vi "数据表比对.vi"(8 "error in (no error)":errorcluster, 9 "查询元素输入":string(combo), 10 "仪器日志参数":string, 11 "table输入":string(combo)) -> (0 "error out":errorcluster, 1 "columns输出":string[](array[string]), 2 "待发送第一条数据":string[](array[string]), 3 "待发送数据":string[][](table))   [LabVIEW 2016, in "数据传输系统-03.lvlib"]
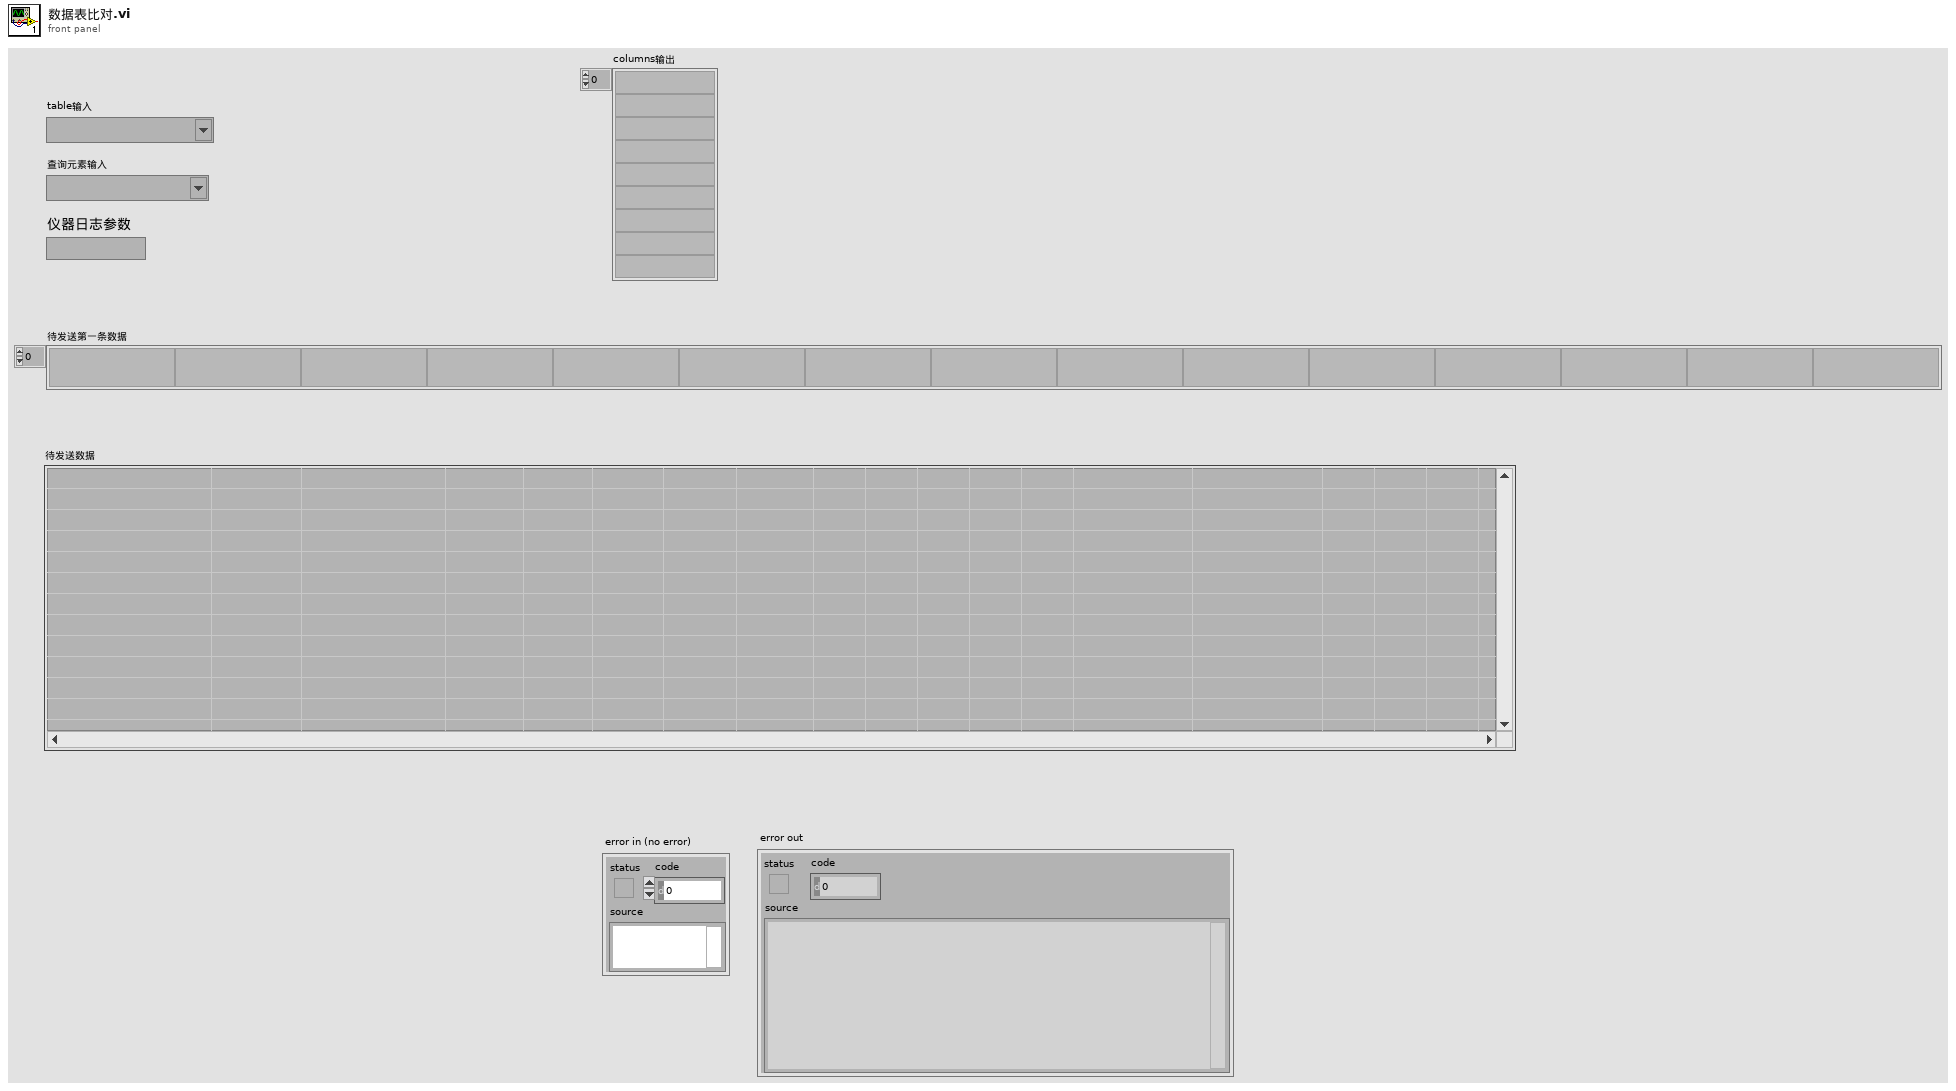
[diagram p1: front panel]
types:
  T1 = cluster{"氨氮仪器日志索引起始时间":string, "总磷仪器日志索引起始时间":string, "总氮仪器日志索引起始时间":string, "CODMn仪器日志索引起始时间":string, "CODCr仪器日志索引起始时间":string, "系统仪器日志索引起始时间":string, "氟化物仪器日志索引起始时间":string, "挥发酚仪器日志索引起始时间":string}
  T2 = cluster{"氨氮仪器参数索引起始时间":string, "总磷仪器参数索引起始时间":string, "总氮仪器参数索引起始时间":string, "CODMn仪器参数索引起始时间":string, "CODCr仪器参数索引起始时间":string, "DO仪器参数索引起始时间":string, "PH仪器参数索引起始时间":string, "比电导率仪器参数索引起始时间":string, "水温仪器参数索引起始时间":string, "浊度仪器参数索引起始时间":string, "叶绿素a仪器参数索引起始时间":string, "藻密度仪器参数索引起始时间":string, "ORP仪器参数索引起始时间":string, "氟化物仪器参数索引起始时间":string, "挥发酚仪器参数索引起始时间":string}
  T3 = typedef "数据传输系统-03.lvlib/应用环境.ctl" = enum16{"STD", "GB212", "婉仪平台"}
  T4 = cluster{"氨氮报警信息索引起始时间":string, "总磷报警信息索引起始时间":string, "总氮报警信息索引起始时间":string, "CODMn报警信息索引起始时间":string, "CODCr报警信息索引起始时间":string, "DO报警信息索引起始时间":string, "PH报警信息索引起始时间":string, "比电导率报警信息索引起始时间":string, "水温报警信息索引起始时间":string, "浊度报警信息索引起始时间":string, "叶绿素报警信息索引起始时间":string, "系统报警信息索引起始时间":string, "氟化物报警信息索引起始时间":string, "挥发酚报警信息索引起始时间":string}
  T5 = cluster{"氨氮零点核查索引起始时间":string, "总磷零点核查索引起始时间":string, "总氮零点核查索引起始时间":string, "CODMn零点核查索引起始时间":string, "CODCr零点核查索引起始时间":string, "亚硝酸盐零点核查索引起始时间":string, "硫化物零点核查索引起始时间":string, "ORP零点核查索引起始时间":string, "氟化物零点核查索引起始时间":string, "挥发酚零点核查索引起始时间":string}
  T6 = cluster{"氨氮标样核查索引起始时间":string, "总磷标样核查索引起始时间":string, "总氮标样核查索引起始时间":string, "CODMn标样核查索引起始时间":string, "CODCr标样核查索引起始时间":string, "DO标样核查索引起始时间":string, "PH标样核查索引起始时间":string, "比电导率标样核查索引起始时间":string, "水温标样核查索引起始时间":string, "浊度标样核查索引起始时间":string, "叶绿素a标样核查索引起始时间":string, "藻密度标样核查索引起始时间":string, "亚硝酸盐标样核查索引起始时间":string, "硫化物标样核查索引起始时间":string, "ORP标样核查索引起始时间":string, "氟化物标样核查索引起始时间":string, "挥发酚标样核查索引起始时间":string, "氯化物标样核查索引起始时间":string}
  T7 = cluster{"氨氮跨度核查索引起始时间":string, "总磷跨度核查索引起始时间":string, "总氮跨度核查索引起始时间":string, "CODMn跨度核查索引起始时间":string, "CODCr跨度核查索引起始时间":string, "亚硝酸盐跨度核查索引起始时间":string, "硫化物跨度核查索引起始时间":string, "ORP跨度核查索引起始时间":string, "氟化物跨度核查索引起始时间":string, "挥发酚跨度核查索引起始时间":string}
  T8 = typedef "LVDateTimeRec.ctl" = cluster{"秒数的小数部分":dbl, "秒":i32, "分":i32, "时":i32, "日":i32, "月":i32, "年":i32, "天数（周）":i32, "天数（年）":i32, "DST":i32}
  T9 = cluster{"氨氮加标回收索引起始时间":string, "总磷加标回收索引起始时间":string, "总氮加标回收索引起始时间":string, "CODMn加标回收索引起始时间":string, "CODCr加标回收索引起始时间":string, "氟化物加标回收索引起始时间":string, "挥发酚加标回收索引起始时间":string}
  T10 = cluster{"氨氮平行样索引起始时间":string, "总磷平行样索引起始时间":string, "总氮平行样索引起始时间":string, "CODMn平行样索引起始时间":string, "CODCr平行样索引起始时间":string, "氟化物平行样索引起始时间":string, "挥发酚平行样索引起始时间":string}
  T11 = cluster{"氨氮集成干预索引起始时间":string, "总磷集成干预索引起始时间":string, "总氮集成干预索引起始时间":string, "CODMn集成干预索引起始时间":string, "CODCr集成干预索引起始时间":string, "DO集成干预索引起始时间":string, "PH集成干预索引起始时间":string, "比电导率集成干预索引起始时间":string, "水温集成干预索引起始时间":string, "浊度集成干预索引起始时间":string, "叶绿素a集成干预索引起始时间":string, "藻密度集成干预索引起始时间":string, "亚硝酸盐集成干预索引起始时间":string, "硫化物集成干预索引起始时间":string, "ORP集成干预索引起始时间":string, "氟化物集成干预索引起始时间":string, "挥发酚集成干预索引起始时间":string, "氯化物集成干预索引起始时间":string}
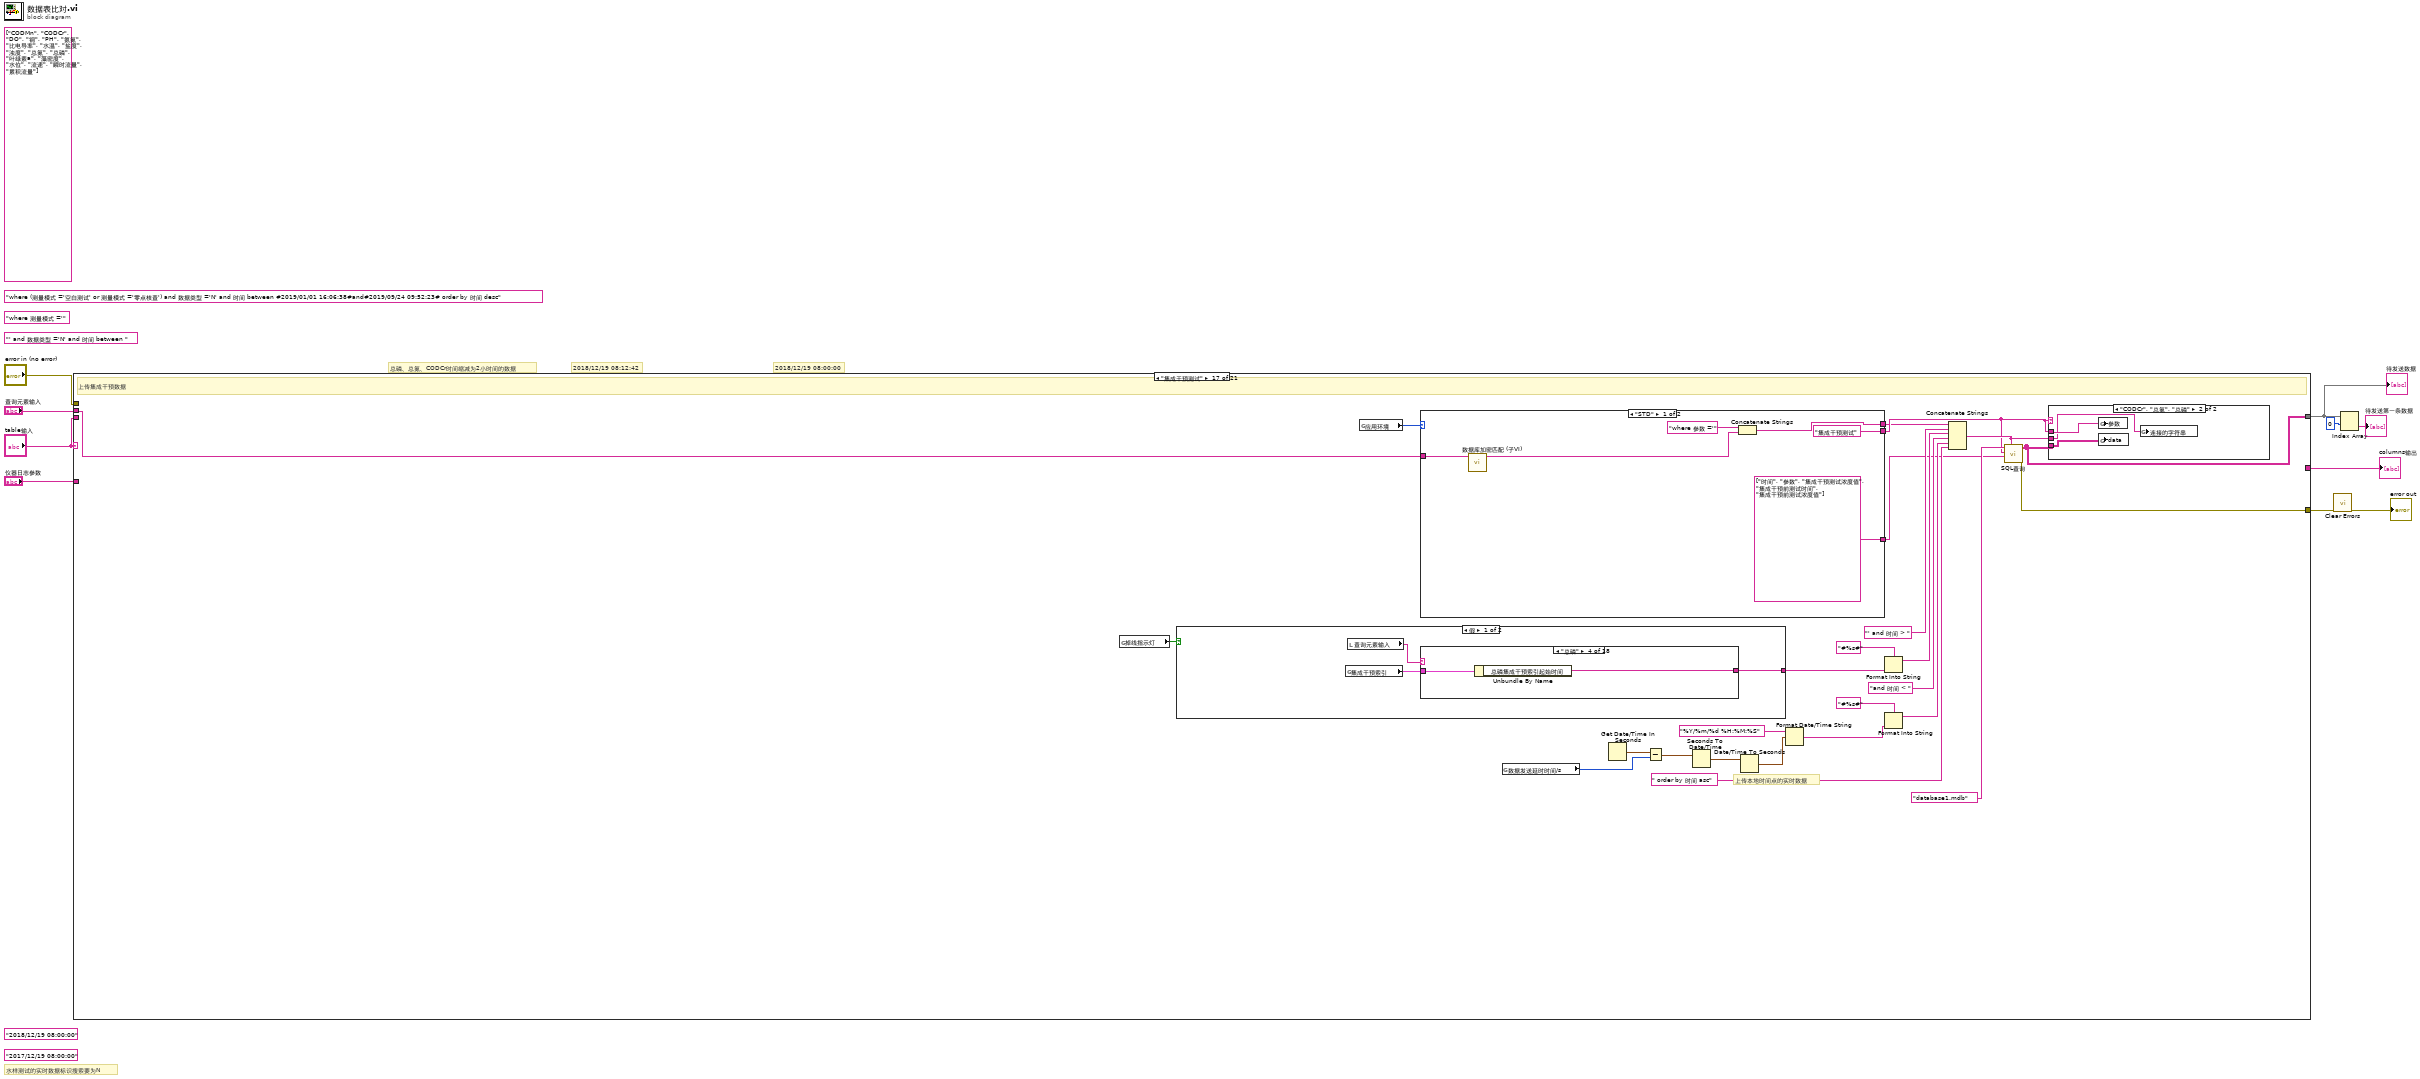
[diagram p0: block diagram]
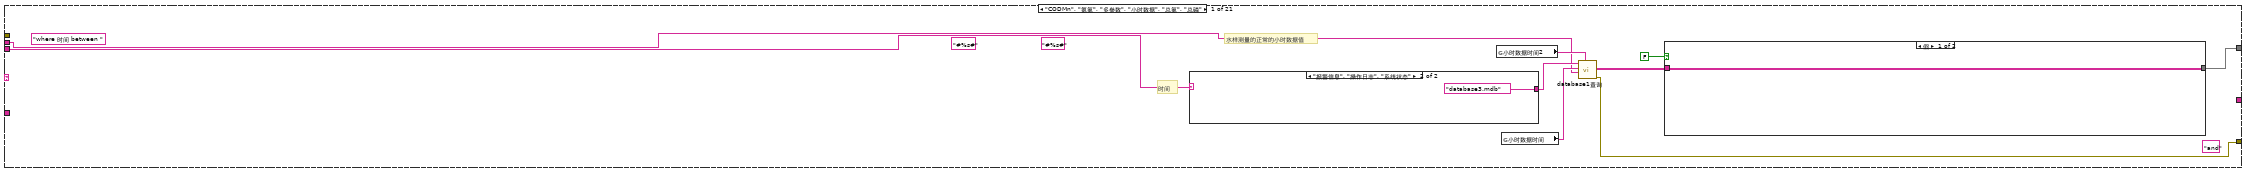
[diagram p2: hidden frame]
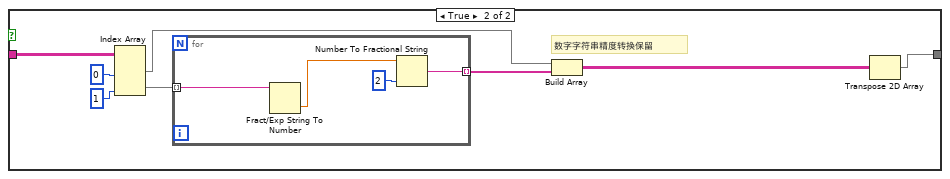
[diagram p3: hidden frame]
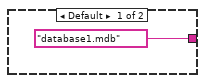
[diagram p4: hidden frame]
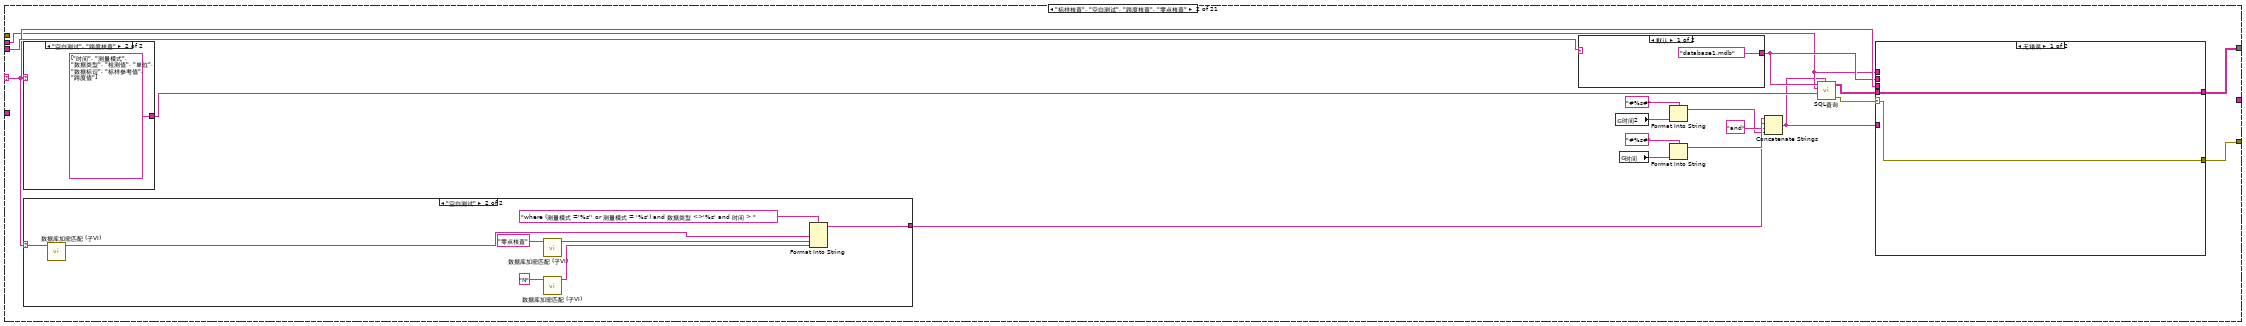
[diagram p5: hidden frame]
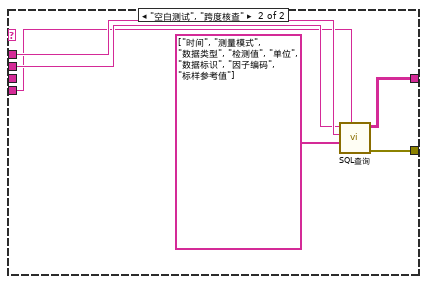
[diagram p7: hidden frame]
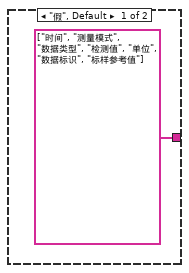
[diagram p8: hidden frame]
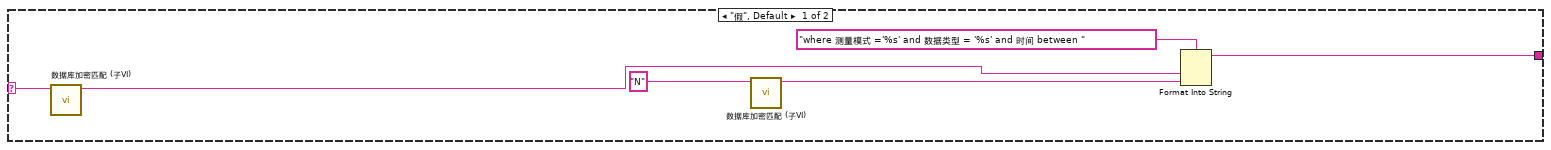
[diagram p9: hidden frame]
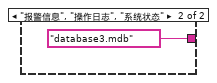
[diagram p10: hidden frame]
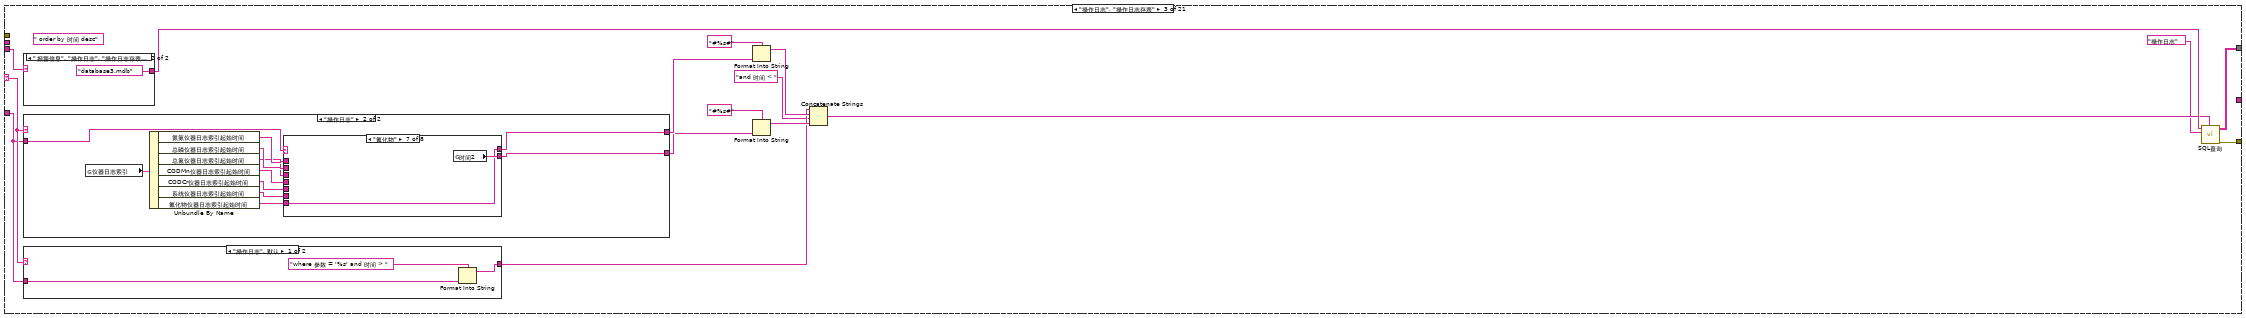
[diagram p11: hidden frame]
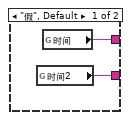
[diagram p12: hidden frame]
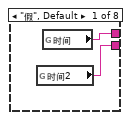
[diagram p13: hidden frame]
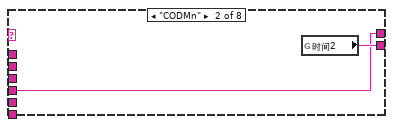
[diagram p14: hidden frame]
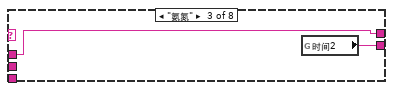
[diagram p15: hidden frame]
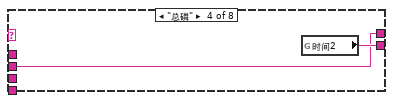
[diagram p16: hidden frame]
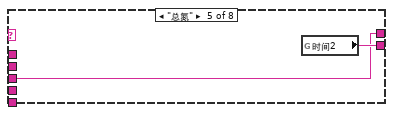
[diagram p17: hidden frame]
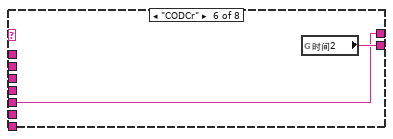
[diagram p18: hidden frame]
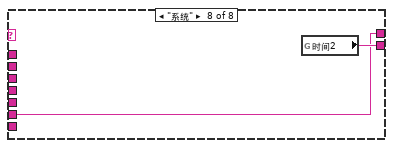
[diagram p19: hidden frame]
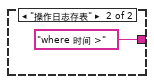
[diagram p20: hidden frame]
diagram:
  (unwired) "' and 数据类型 ='N' and 时间 between "
  (unwired) "where 测量模式 ='" ("condition")
  (unwired) "where (测量模式 ='空白测试' or 测量模式 ='零点核查') and 数据类型 ='N' and 时间 between #2019/01/01 16:06:38#and#2019/09/24 09:52:23# order by 时间 desc" ("condition")
  (unwired) string[] ["CODMn", "CODCr", "DO", "铜", "PH", "氨氮", "比电导率", "水温", "盐度", "浊度", "总氮", "总磷", "叶绿素a", "藻密度", "水位", "流速", "瞬时流量", "累积流量"] ("查询参数数组")
  (unwired) "2017/12/19 08:00:00"
  (unwired) "2018/12/19 08:00:00"
  # "水样测试的实时数据标识搜索要为N"
  # "2018/12/19 08:00:00"
  # "总磷、总氮、CODCr时间缩减为2小时间的数据"
  # "2018/12/19 08:12:42"
  n1 = case shown="\"集成干预测试\"" "table输入" {
    selector: "table输入" -> [_ w41 w91 _ _ _ _ _ _ w389 _ _ _ _ _ _ _ _ _ _ _]
    tunnel: "error in (no error)" -> [_ _ _ _ _ _ _ _ _ _ _ _ w517 _ _ _ _ _ _ _ _]
    tunnel: [w17 w35 w100 w153 w173 w192 w201 w260 w364 w403 w495 w514 w517 w518 w717 w764 w831 w902 w944 w987 w1038] -> w8
    tunnel: [w13 w36 w98 w151 w171 w190 w228 w262 w356 w401 w479 w513 w515 w520 w715 w767 w829 w905 w947 w990 w1040] -> w1
    tunnel: "table输入" -> [w19 w52 w102 _ _ _ w200 w263 _ w393 _ w510 _ _ _ _ _ _ _ _ _]
    tunnel: "查询元素输入" -> [w11 w39 _ _ _ _ _ _ _ _ _ _ _ w524 w702 w749 w817 w894 w936 w977 w1034]
    tunnel: "仪器日志参数" -> [_ _ w88 _ _ w178 w195 w251 w335 w388 w478 _ _ _ _ _ _ _ _ _ _]
    tunnel: [_ _ _ _ _ _ _ _ _ _ _ w509 _ _ _ _ _ _ _ _ _] -> w2
    frame "CODMn", "氨氮", "多参数", "小时数据", "总氮", "总磷" {
      (unwired) "and" ("字符串")
      (unwired) "#%s#" ("初始字符串")
      (unwired) "#%s#" ("初始字符串")
      (unwired) "where 时间 between " ("condition")
      # "水样测量的正常的小时数据值"
      # "时间"
      n2 = case shown="\"报警信息\", \"操作日志\", \"系统状态\"" w19 {
        tunnel: ["database1.mdb" ("database") "database3.mdb" ("database")] -> w18
        frame Default {
        }
        frame "报警信息", "操作日志", "系统状态" {
        }
      }
      n3 = global read "全局 时间2.vi" "小时数据时间2"() -> (w15:string)
      n4 = global read "全局 水样时间.vi" "小时数据时间"() -> (w16:string)
      n5 = call "database1查询.vi"("时间2"=w15, "table"=w11, "时间1"=w16, "database"=w18) -> ("error out"=w17:errorcluster, "data"=w14:string[][])  [unwired: 3 in, 2 out]
      n6 = case shown="假" FALSE {
        tunnel: w14 -> [w20 w28]
        tunnel: [w20 w21] -> w13
        frame False {
        }
        frame True {
          # "数字字符串精度转换保留"
          n7 = Index Array(array=w28, index (col) #1=0 ("禁用的索引 (列)"), index (col) #2=1 ("索引 (列)")) -> (element #1=w24:string[], element #2=w25:string[])  [unwired: 2 in]
          n8 = for {
            tunnel: w25 -> [w30] mode=indexing
            tunnel: [w29] -> w23 mode=indexing
            n9 = Fract/Exp String To Number(string=w30) -> (number=w31:dbl)  [unwired: 3 in, 1 out]
            n10 = Number To Fractional String(number=w31, precision (6)=i16 2 ("精度(6)")) -> (F-format string=w29:string)  [unwired: 2 in]
          }
          n11 = Build Array(w24, w23) -> (w22:string[][])
          n12 = Transpose 2D Array(2D array=w22) -> (transposed array=w21:string[][])
        }
      }
    }
    frame "标样核查", "空白测试", "跨度核查", "零点核查" {
      n13 = case shown="\"空白测试\", \"跨度核查\"" w41 {
        tunnel: [string[] ["时间", "测量模式", "数据类型", "检测值", "单位", "数据标识", "标样参考值"] ("columns") string[] ["时间", "测量模式", "数据类型", "检测值", "单位", "数据标识", "标样参考值", "跨度值"] ("columns")] -> w43
        frame "假", Default {
        }
        frame "空白测试", "跨度核查" {
        }
      }
      n14 = case shown="\"空白测试\"" w41 {
        selector: w41 -> [w74 w81]
        tunnel: [w75 w83] -> w44
        frame "假", Default {
          n15 = call "数据库加密匹配 (子VI).vi"("输入参数"=w74) -> ("Encoded String"=w73:string)  [unwired: 10 in]
          n16 = call "数据库加密匹配 (子VI).vi"("输入参数"="N" ("字符串")) -> ("Encoded String"=w71:string)  [unwired: 10 in]
          n17 = Format Into String(format string="where 测量模式 ='%s' and 数据类型 = '%s' and 时间 between " ("格式字符串"), w73, w71) -> (resulting string=w75:string)  [unwired: 2 in, 1 out]
        }
        frame "空白测试" {
          n18 = call "数据库加密匹配 (子VI).vi"("输入参数"=w81) -> ("Encoded String"=w82:string)  [unwired: 10 in]
          n19 = call "数据库加密匹配 (子VI).vi"("输入参数"="零点核查") -> ("Encoded String"=w79:string)  [unwired: 10 in]
          n20 = call "数据库加密匹配 (子VI).vi"("输入参数"="N") -> ("Encoded String"=w77:string)  [unwired: 10 in]
          n21 = Format Into String(format string="where (测量模式 ='%s'' or 测量模式 = '%s') and 数据类型 <>'%s' and 时间 > " ("格式字符串"), w82, w79, w77) -> (resulting string=w83:string)  [unwired: 2 in, 1 out]
        }
      }
      n22 = case shown="默认" w52 {
        tunnel: ["database1.mdb" ("database") "database3.mdb" ("database")] -> w40
        frame Default {
        }
        frame "报警信息", "操作日志", "系统状态" {
        }
      }
      n23 = global read "全局 时间2.vi" "时间2"() -> (w45:string)
      n24 = global read "全局 水样时间.vi" "时间"() -> (w46:string)
      n25 = Format Into String(format string="#%s#" ("初始字符串"), w45) -> (resulting string=w47:string)  [unwired: 2 in, 1 out]
      n26 = Format Into String(format string="#%s#" ("初始字符串"), w46) -> (resulting string=w51:string)  [unwired: 2 in, 1 out]
      n27 = Concatenate Strings(w44, w51, "and" ("字符串"), w47) -> (w38:string)
      n28 = call "SQL查询.vi"("condition"=w38, "columns"=w43, "table输入"=w39, "database"=w40) -> ("error out"=w42:errorcluster, "data"=w37:string[][])  [unwired: 4 in, 2 out]
      n29 = case shown="无错误" w42 {
        selector: w42 -> [w53 _]
        tunnel: w41 -> [_ w61]
        tunnel: w39 -> [_ w60]
        tunnel: w40 -> [_ w59]
        tunnel: w38 -> [_ w58]
        tunnel: w37 -> [w54 w56]
        tunnel: [w54 w57] -> w36
        tunnel: [w53 w55] -> w35
        frame No Error {
        }
        frame Error {
          # "兼容旧数据库没有跨度值版本"
          n30 = case shown="\"假\", 默认" w61 {
            tunnel: w60 -> [_ w67]
            tunnel: w59 -> [_ w66]
            tunnel: w58 -> [_ w65]
            tunnel: [w62 w64] -> w57
            tunnel: w56 -> [w62 _]
            tunnel: [_ w63] -> w55
            frame "假", Default {
            }
            frame "空白测试", "跨度核查" {
              n31 = call "SQL查询.vi"("condition"=w65, "columns"=string[] ["时间", "测量模式", "数据类型", "检测值", "单位", "数据标识", "因子编码", "标样参考值"], "table输入"=w67, "database"=w66) -> ("error out"=w63:errorcluster, "data"=w64:string[][])  [unwired: 4 in, 2 out]
            }
          }
        }
      }
    }
    frame "操作日志", "操作日志存表" {
      (unwired) " order by 时间 desc" ("字符串")
      n32 = case shown="\"报警信息\", \"操作日志\", \"操作日志存表\", \"系统状态\"" w102 {
        tunnel: ["database1.mdb" ("database") "database3.mdb" ("database")] -> w101
        frame Default {
        }
        frame "报警信息", "操作日志", "操作日志存表", "系统状态" {
        }
      }
      n33 = case shown="\"操作日志\"" w91 {
        tunnel: [w104 w114] -> w90
        tunnel: [w103 w106] -> w89
        tunnel: w88 -> [_ w115]
        frame "假", Default {
          n34 = global read "全局 时间2.vi" "时间2"() -> (w103:string)
          n35 = global read "全局 水样时间.vi" "时间"() -> (w104:string)
        }
        frame "操作日志" {
          n36 = global read "全局 时间2.vi" "仪器日志索引"() -> (w113:T1)
          n37 = Unbundle By Name(w113) -> ("氨氮仪器日志索引起始时间"=w112:string, "总磷仪器日志索引起始时间"=w111:string, "总氮仪器日志索引起始时间"=w110:string, "CODMn仪器日志索引起始时间"=w109:string, "CODCr仪器日志索引起始时间"=w108:string, "系统仪器日志索引起始时间"=w107:string, "氟化物仪器日志索引起始时间"=w105:string)
          n38 = case shown="\"氟化物\"" w115 {
            tunnel: [w116 w119 w121 w123 w125 w127 w129 w131] -> w106
            tunnel: [w117 w118 w120 w122 w124 w126 w128 w130] -> w114
            tunnel: w112 -> [_ _ w120 _ _ _ _ _]
            tunnel: w111 -> [_ _ _ w122 _ _ _ _]
            tunnel: w110 -> [_ _ _ _ w124 _ _ _]
            tunnel: w109 -> [_ w118 _ _ _ _ _ _]
            tunnel: w108 -> [_ _ _ _ _ w126 _ _]
            tunnel: w107 -> [_ _ _ _ _ _ _ w130]
            tunnel: w105 -> [_ _ _ _ _ _ w128 _]
            frame "假", Default {
              n39 = global read "全局 时间2.vi" "时间2"() -> (w116:string)
              n40 = global read "全局 水样时间.vi" "时间"() -> (w117:string)
            }
            frame "CODMn" {
              n41 = global read "全局 时间2.vi" "时间2"() -> (w119:string)
            }
            frame "氨氮" {
              n42 = global read "全局 时间2.vi" "时间2"() -> (w121:string)
            }
            frame "总磷" {
              n43 = global read "全局 时间2.vi" "时间2"() -> (w123:string)
            }
            frame "总氮" {
              n44 = global read "全局 时间2.vi" "时间2"() -> (w125:string)
            }
            frame "CODCr" {
              n45 = global read "全局 时间2.vi" "时间2"() -> (w127:string)
            }
            frame "氟化物" {
              n46 = global read "全局 时间2.vi" "时间2"() -> (w129:string)
            }
            frame "系统" {
              n47 = global read "全局 时间2.vi" "时间2"() -> (w131:string)
            }
          }
        }
      }
      n48 = case shown="\"操作日志\", 默认" w91 {
        tunnel: [w133 "where 时间 >" ("condition")] -> w93
        tunnel: w88 -> [w132 _]
        frame "操作日志", Default {
          n49 = Format Into String(format string="where 参数 = '%s' and 时间 > " ("condition"), w132) -> (resulting string=w133:string)  [unwired: 2 in, 1 out]
        }
        frame "操作日志存表" {
        }
      }
      n50 = Format Into String(format string="#%s#" ("初始字符串"), w90) -> (resulting string=w97:string)  [unwired: 2 in, 1 out]
      n51 = Format Into String(format string="#%s#" ("初始字符串"), w89) -> (resulting string=w94:string)  [unwired: 2 in, 1 out]
      n52 = Concatenate Strings(w93, w97, "and 时间 < " ("字符串"), w94) -> (w99:string)
      n53 = call "SQL查询.vi"("condition"=w99, "table输入"="操作日志", "database"=w101) -> ("error out"=w100:errorcluster, "data"=w98:string[][])  [unwired: 5 in, 2 out]
    }
    frame "3092日志信息" {
      n54 = global read "断电保存全局.vi" "日志信息重发"() -> (w138:bool)
      n55 = case shown="真" w138 {
        tunnel: [w155 w156] -> w141
        frame False {
          n56 = Get Date/Time In Seconds() -> (seconds since 1Jan1904=w155:timestamp)
        }
        frame True {
          n57 = global read "断电保存全局.vi" "数据重发结束时间"() -> (w156:timestamp)
        }
      }
      n58 = global read "全局 时间2.vi" "3092日志索引起始时间"() -> (w143:string)
      n59 = Format Date/Time String(time format string (%c)="%Y/%m/%d %H:%M:%S" ("时间格式字符串(%c)"), seconds (now)=w141) -> (date/time string=w140:string)  [unwired: 1 in]
      n60 = Format Into String(format string="#%s#" ("初始字符串"), w143) -> (resulting string=w150:string)  [unwired: 2 in, 1 out]
      n61 = Format Into String(format string="#%s#" ("初始字符串"), w140) -> (resulting string=w147:string)  [unwired: 2 in, 1 out]
      n62 = Concatenate Strings("where 时间 >" ("condition"), w150, "and 时间 < " ("字符串"), w147, " order by 时间 asc" ("字符串")) -> (w152:string)
      n63 = call "SQL查询.vi"("condition"=w152, "table输入"="操作日志", "database"="database3.mdb") -> ("error out"=w153:errorcluster, "data"=w151:string[][])  [unwired: 5 in, 2 out]
    }
    frame "3093报警信息" {
      n64 = global read "断电保存全局.vi" "日志信息重发"() -> (w158:bool)
      n65 = case shown="真" w158 {
        tunnel: [w175 w176] -> w157
        frame False {
          n66 = Get Date/Time In Seconds() -> (seconds since 1Jan1904=w175:timestamp)
        }
        frame True {
          n67 = global read "断电保存全局.vi" "数据重发结束时间"() -> (w176:timestamp)
        }
      }
      n68 = global read "全局 时间2.vi" "3093报警索引起始时间"() -> (w163:string)
      n69 = Format Date/Time String(time format string (%c)="%Y/%m/%d %H:%M:%S" ("时间格式字符串(%c)"), seconds (now)=w157) -> (date/time string=w161:string)  [unwired: 1 in]
      n70 = Format Into String(format string="#%s#" ("初始字符串"), w163) -> (resulting string=w170:string)  [unwired: 2 in, 1 out]
      n71 = Format Into String(format string="#%s#" ("初始字符串"), w161) -> (resulting string=w167:string)  [unwired: 2 in, 1 out]
      n72 = Concatenate Strings("where 时间 >" ("condition"), w170, "and 时间 < " ("字符串"), w167, " order by 时间 asc" ("字符串")) -> (w172:string)
      n73 = call "SQL查询.vi"("condition"=w172, "columns"=string[] ["时间", "参数", "故障现象", "故障分析", "platform_alarm_code", "state"], "table输入"="报警信息", "database"="database3.mdb") -> ("error out"=w173:errorcluster, "data"=w171:string[][])  [unwired: 4 in, 2 out]
    }
    frame "提取操作日志" {
      n74 = call "数据库加密匹配 (子VI).vi"("输入参数"=w178) -> ("Encoded String"=w177:string)  [unwired: 10 in]
      n75 = global read "全局 时间2.vi" "时间2"() -> (w181:string)
      n76 = global read "全局 水样时间.vi" "时间"() -> (w182:string)
      n77 = Format Into String(format string="where 参数 = '%s' and 时间 between" ("condition"), w177) -> (resulting string=w184:string)  [unwired: 2 in, 1 out]
      n78 = Format Into String(format string="#%s#" ("初始字符串"), w182) -> (resulting string=w189:string)  [unwired: 2 in, 1 out]
      n79 = Format Into String(format string="#%s#" ("初始字符串"), w181) -> (resulting string=w185:string)  [unwired: 2 in, 1 out]
      n80 = Concatenate Strings(w184, w189, "and" ("字符串"), w185) -> (w191:string)
      n81 = call "SQL查询.vi"("condition"=w191, "table输入"="操作日志", "database"="database3.mdb") -> ("error out"=w192:errorcluster, "data"=w190:string[][])  [unwired: 5 in, 2 out]
    }
    frame "3090仪器参数" {
      (unwired) string[] ["时间", "参数", "测量量程", "测量精度", "测量间隔", "消解温度", "消解时长", "空白校准时间", "曲线截距", "曲线斜率", "测量检出限", "测量信号值", "线性相关系数", "二次多项式系数", "标样校准时间", "稀释倍数", "三项式系数", "空白标定系数", "量程系数", "F0/ORPA", "F1/ORPB", "F2/ORPK", "F3", "F4", "F5", "F6", "F7", "X0/滴定数", "量程"] ("columns输出")
      n82 = case shown="\"3090仪器参数\"" w200 {
        tunnel: [w231 w232] -> w216
        frame "3090仪器参数" {
          n83 = global read "全局 时间2.vi" "3090仪器参数索引"() -> (w231:T2)
        }
        frame "仪器参数", Default {
          n84 = global read "全局 时间2.vi" "仪器参数索引"() -> (w232:T2)
        }
      }
      n85 = call "数据库加密匹配 (子VI).vi"("输入参数"=w195) -> ("Encoded String"=w194:string)  [unwired: 10 in]
      n86 = global read "断电保存全局.vi" "数据发送延时时间/s"() -> (w197:i32)
      n87 = Unbundle By Name(w216) -> ("氨氮仪器参数索引起始时间"=w215:string, "总磷仪器参数索引起始时间"=w214:string, "总氮仪器参数索引起始时间"=w213:string, "CODMn仪器参数索引起始时间"=w212:string, "CODCr仪器参数索引起始时间"=w211:string, "DO仪器参数索引起始时间"=w209:string, "PH仪器参数索引起始时间"=w208:string, "比电导率仪器参数索引起始时间"=w207:string, "水温仪器参数索引起始时间"=w206:string, "浊度仪器参数索引起始时间"=w205:string, "叶绿素a仪器参数索引起始时间"=w204:string, "藻密度仪器参数索引起始时间"=w203:string, "ORP仪器参数索引起始时间"=w202:string, "氟化物仪器参数索引起始时间"=w193:string)
      n88 = Format Into String(format string="where 参数 = '%s' and 时间 > " ("condition"), w194) -> (resulting string=w223:string)  [unwired: 2 in, 1 out]
      n89 = Get Date/Time In Seconds() -> (seconds since 1Jan1904=w198:timestamp)
      n90 = case shown="\"氟化物\"" w195 {
        tunnel: w215 -> [_ _ w235 _ _ _ _ _ _ _ _ _ _ _ _]
        tunnel: w214 -> [_ _ _ w236 _ _ _ _ _ _ _ _ _ _ _]
        tunnel: w213 -> [_ _ _ _ w237 _ _ _ _ _ _ _ _ _ _]
        tunnel: w212 -> [w233 w234 _ _ _ _ _ _ _ _ _ _ _ _ _]
        tunnel: w211 -> [_ _ _ _ _ w238 _ _ _ _ _ _ _ _ _]
        tunnel: [w233 w234 w235 w236 w237 w238 w239 w240 w241 w242 w243 w244 w245 w246 w247] -> w210
        tunnel: w209 -> [_ _ _ _ _ _ w239 _ _ _ _ _ _ _ _]
        tunnel: w208 -> [_ _ _ _ _ _ _ w240 _ _ _ _ _ _ _]
        tunnel: w207 -> [_ _ _ _ _ _ _ _ w241 _ _ _ _ _ _]
        tunnel: w206 -> [_ _ _ _ _ _ _ _ _ w242 _ _ _ _ _]
        tunnel: w205 -> [_ _ _ _ _ _ _ _ _ _ w243 _ _ _ _]
        tunnel: w204 -> [_ _ _ _ _ _ _ _ _ _ _ w244 _ _ _]
        tunnel: w203 -> [_ _ _ _ _ _ _ _ _ _ _ _ w245 _ _]
        tunnel: w202 -> [_ _ _ _ _ _ _ _ _ _ _ _ _ w246 _]
        tunnel: w193 -> [_ _ _ _ _ _ _ _ _ _ _ _ _ _ w247]
        frame "假", Default {
        }
        frame "CODMn" {
        }
        frame "氨氮" {
        }
        frame "总磷" {
        }
        frame "总氮" {
        }
        frame "CODCr" {
        }
        frame "溶解氧" {
        }
        frame "PH" {
        }
        frame "电导率" {
        }
        frame "水温" {
        }
        frame "浊度" {
        }
        frame "叶绿素" {
        }
        frame "藻密度" {
        }
        frame "ORP" {
        }
        frame "氟化物" {
        }
      }
      n91 = Subtract(x=w198, y=w197) -> (x-y=w196:timestamp)
      n92 = Format Date/Time String(time format string (%c)="%Y/%m/%d %H:%M:%S" ("时间格式字符串(%c)"), seconds (now)=w196) -> (date/time string=w219:string)  [unwired: 1 in]
      n93 = Search and Replace String(input string=w219, search string="." ("搜索字符串")) -> (result string=w217:string)  [unwired: 6 in, 3 out]
      n94 = Format Into String(format string="#%s#" ("初始字符串"), w217) -> (resulting string=w224:string)  [unwired: 2 in, 1 out]
      n95 = Format Into String(format string="#%s#" ("初始字符串"), w210) -> (resulting string=w227:string)  [unwired: 2 in, 1 out]
      n96 = Concatenate Strings(w223, w227, "and 时间 < " ("字符串"), w224, " order by 时间 asc" ("字符串")) -> (w229:string)
      n97 = call "SQL查询.vi"("condition"=w229, "table输入"=w200, "database"="database3.mdb") -> ("error out"=w201:errorcluster, "data"=w228:string[][])  [unwired: 5 in, 2 out]
    }
    frame "仪器参数" {
      n98 = case shown="\"仪器参数\", 默认" w263 {
        tunnel: [w318 w319] -> w280
        frame "3090仪器参数" {
          n99 = global read "全局 时间2.vi" "3090仪器参数索引"() -> (w318:T2)
        }
        frame "仪器参数", Default {
          n100 = global read "全局 时间2.vi" "仪器参数索引"() -> (w319:T2)
        }
      }
      n101 = global read "断电保存全局.vi" "应用环境"() -> (w253:T3)
      n102 = case shown="\"GB212\", 默认" w253 {
        tunnel: [w296 string[] ["时间", "数据类型", "测量量程", "测量精度", "测量间隔", "消解温度", "消解时长", "空白校准时间", "曲线截距", "曲线斜率", "测量检出限", "测量信号值", "线性相关系数", "二次多项式系数", "标样校准时间"] ("columns输出")] -> w266
        tunnel: w251 -> [w295 _]
        frame "STD" {
          n103 = case shown="\"CODMn\"" w295 {
            tunnel: [string[] ["时间", "数据类型", "测量量程", "测量精度", "测量间隔", "消解温度", "消解时长", "空白校准时间", "曲线截距", "曲线斜率", "测量检出限", "测量信号值", "线性相关系数", "二次多项式系数", "标样校准时间", "量程"] ("columns输出") string[] ["时间", "数据类型", "测量量程", "测量精度", "测量间隔", "消解温度", "消解时长", "空白校准时间", "曲线截距", "曲线斜率", "测量检出限", "测量信号值", "线性相关系数", "二次多项式系数", "标样校准时间", "量程标识"] ("columns输出")] -> w296
            frame "CODMn" {
            }
            frame "", Default {
            }
          }
        }
        frame "GB212", Default {
        }
      }
      n104 = Unbundle By Name(w280) -> ("氨氮仪器参数索引起始时间"=w279:string, "总磷仪器参数索引起始时间"=w278:string, "总氮仪器参数索引起始时间"=w277:string, "CODMn仪器参数索引起始时间"=w276:string, "CODCr仪器参数索引起始时间"=w275:string, "DO仪器参数索引起始时间"=w274:string, "PH仪器参数索引起始时间"=w273:string, "比电导率仪器参数索引起始时间"=w272:string, "水温仪器参数索引起始时间"=w271:string, "浊度仪器参数索引起始时间"=w270:string, "叶绿素a仪器参数索引起始时间"=w269:string, "藻密度仪器参数索引起始时间"=w268:string, "ORP仪器参数索引起始时间"=w267:string, "氟化物仪器参数索引起始时间"=w248:string)
      n105 = case shown="\"氟化物\"" w251 {
        tunnel: w279 -> [_ _ w322 _ _ _ _ _ _ _ _ _ _ _ _]
        tunnel: w278 -> [_ _ _ w323 _ _ _ _ _ _ _ _ _ _ _]
        tunnel: w277 -> [_ _ _ _ w324 _ _ _ _ _ _ _ _ _ _]
        tunnel: w276 -> [w320 w321 _ _ _ _ _ _ _ _ _ _ _ _ _]
        tunnel: w275 -> [_ _ _ _ _ w325 _ _ _ _ _ _ _ _ _]
        tunnel: [w320 w321 w322 w323 w324 w325 w326 w327 w328 w329 w330 w331 w332 w333 w334] -> w265
        tunnel: w274 -> [_ _ _ _ _ _ w326 _ _ _ _ _ _ _ _]
        tunnel: w273 -> [_ _ _ _ _ _ _ w327 _ _ _ _ _ _ _]
        tunnel: w272 -> [_ _ _ _ _ _ _ _ w328 _ _ _ _ _ _]
        tunnel: w271 -> [_ _ _ _ _ _ _ _ _ w329 _ _ _ _ _]
        tunnel: w270 -> [_ _ _ _ _ _ _ _ _ _ w330 _ _ _ _]
        tunnel: w269 -> [_ _ _ _ _ _ _ _ _ _ _ w331 _ _ _]
        tunnel: w268 -> [_ _ _ _ _ _ _ _ _ _ _ _ w332 _ _]
        tunnel: w267 -> [_ _ _ _ _ _ _ _ _ _ _ _ _ w333 _]
        tunnel: w248 -> [_ _ _ _ _ _ _ _ _ _ _ _ _ _ w334]
        frame "假", Default {
        }
        frame "CODMn" {
        }
        frame "氨氮" {
        }
        frame "总磷" {
        }
        frame "总氮" {
        }
        frame "CODCr" {
        }
        frame "溶解氧" {
        }
        frame "PH" {
        }
        frame "电导率" {
        }
        frame "水温" {
        }
        frame "浊度" {
        }
        frame "叶绿素" {
        }
        frame "藻密度" {
        }
        frame "ORP" {
        }
        frame "氟化物" {
        }
      }
      n106 = global read "断电保存全局.vi" "日志信息重发"() -> (w250:bool)
      n107 = case shown="假" w250 {
        tunnel: [w291 w294] -> w249
        frame False {
          n108 = global read "断电保存全局.vi" "数据发送延时时间/s"() -> (w292:i32)
          n109 = Get Date/Time In Seconds() -> (seconds since 1Jan1904=w293:timestamp)
          n110 = Subtract(x=w293, y=w292) -> (x-y=w291:timestamp)
        }
        frame True {
          n111 = global read "断电保存全局.vi" "数据重发结束时间"() -> (w294:timestamp)
        }
      }
      n112 = Format Into String(format string="#%s#" ("初始字符串"), w265) -> (resulting string=w288:string)  [unwired: 2 in, 1 out]
      n113 = call "数据库加密匹配 (子VI).vi"("输入参数"="N") -> ("Encoded String"=w254:string)  [unwired: 10 in]
      n114 = Format Date/Time String(time format string (%c)="%Y/%m/%d %H:%M:%S" ("时间格式字符串(%c)"), seconds (now)=w249) -> (date/time string=w282:string)  [unwired: 1 in]
      n115 = Search and Replace String(input string=w282, search string="." ("搜索字符串")) -> (result string=w264:string)  [unwired: 6 in, 3 out]
      n116 = Format Into String(format string="where 数据类型 = '%s' and 时间 > " ("condition"), w254) -> (resulting string=w256:string)  [unwired: 2 in, 1 out]
      n117 = Format Into String(format string="#%s#" ("初始字符串"), w264) -> (resulting string=w285:string)  [unwired: 2 in, 1 out]
      n118 = Concatenate Strings(w256, w288, "and 时间 < " ("字符串"), w285, " order by 时间 asc" ("字符串")) -> (w289:string)
      n119 = call "SQL查询.vi"("condition"=w289, "columns"=w266, "table输入"=w251, "database"="database1.mdb") -> ("error out"=w259:errorcluster, "data"=w261:string[][])  [unwired: 4 in, 2 out]
      n120 = Empty Array?(array=w261) -> ()  [unwired: 1 out]
      n121 = case shown="假" FALSE {
        tunnel: w251 -> [_ w315]
        tunnel: w265 -> [_ w311]
        tunnel: w264 -> [_ w307]
        tunnel: w263 -> [_ w304]
        tunnel: [w301 w303] -> w262
        tunnel: w261 -> [w301 _]
        tunnel: [w300 w302] -> w260
        tunnel: w259 -> [w300 _]
        frame False {
        }
        frame True {
          n122 = Format Into String(format string="#%s#" ("初始字符串"), w311) -> (resulting string=w310:string)  [unwired: 2 in, 1 out]
          n123 = Format Into String(format string="#%s#" ("初始字符串"), w307) -> (resulting string=w306:string)  [unwired: 2 in, 1 out]
          n124 = Format Into String(format string="where 参数 = '%s' and 时间 between" ("condition"), w315) -> (resulting string=w313:string)  [unwired: 2 in, 1 out]
          n125 = Concatenate Strings(w313, w310, "and" ("字符串"), w306, " order by 时间 asc" ("字符串")) -> (w314:string)
          n126 = call "SQL查询.vi"("condition"=w314, "table输入"=w304, "database"="database3.mdb") -> ("error out"=w302:errorcluster, "data"=w303:string[][])  [unwired: 5 in, 2 out]
        }
      }
    }
    frame "提取仪器参数" {
      w358 = 0 ("索引 (行)")
      n127 = call "数据库加密匹配 (子VI).vi"("输入参数"=w335) -> ("Encoded String"=w338:string)  [unwired: 10 in]
      n128 = global read "断电保存全局.vi" "应用环境"() -> (w336:T3)
      n129 = case shown="\"GB212\", 默认" w336 {
        tunnel: [w366 string[] ["时间", "数据类型", "测量量程", "测量精度", "测量间隔", "消解温度", "消解时长", "空白校准时间", "曲线截距", "曲线斜率", "测量检出限", "测量信号值", "线性相关系数", "二次多项式系数", "标样校准时间"] ("columns输出")] -> w337
        tunnel: w335 -> [w365 _]
        frame "STD" {
          n130 = case shown="\"CODMn\"" w365 {
            tunnel: [string[] ["时间", "数据类型", "测量量程", "测量精度", "测量间隔", "消解温度", "消解时长", "空白校准时间", "曲线截距", "曲线斜率", "测量检出限", "测量信号值", "线性相关系数", "二次多项式系数", "标样校准时间", "量程"] ("columns输出") string[] ["时间", "数据类型", "测量量程", "测量精度", "测量间隔", "消解温度", "消解时长", "空白校准时间", "曲线截距", "曲线斜率", "测量检出限", "测量信号值", "线性相关系数", "二次多项式系数", "标样校准时间", "量程标识"] ("columns输出")] -> w366
            frame "CODMn" {
            }
            frame "", Default {
            }
          }
        }
        frame "GB212", Default {
        }
      }
      n131 = call "数据库加密匹配 (子VI).vi"("输入参数"="N") -> ("Encoded String"=w340:string)  [unwired: 10 in]
      n132 = global read "全局 时间2.vi" "时间2"() -> (w349:string)
      n133 = global read "全局 水样时间.vi" "时间"() -> (w347:string)
      n134 = Format Into String(format string="where 数据类型 = '%s' and 时间 between" ("condition"), w340) -> (resulting string=w341:string)  [unwired: 2 in, 1 out]
      n135 = Format Into String(format string="#%s#" ("初始字符串"), w347) -> (resulting string=w354:string)  [unwired: 2 in, 1 out]
      n136 = Format Into String(format string="#%s#" ("初始字符串"), w349) -> (resulting string=w350:string)  [unwired: 2 in, 1 out]
      n137 = Concatenate Strings(w341, w354, "and" ("字符串"), w350, " order by 时间 desc" ("字符串")) -> (w346:string)
      n138 = call "SQL查询.vi"("condition"=w346, "columns"=w337, "table输入"=w335, "database"="database1.mdb") -> ("error out"=w343:errorcluster, "data"=w344:string[][])  [unwired: 4 in, 2 out]
      n139 = Empty Array?(array=w344) -> (empty?=w345:bool)
      n140 = case shown="真" w345 {
        tunnel: [w370 w386] -> w364
        tunnel: w338 -> [_ w374]
        tunnel: [w371 w372] -> w363
        tunnel: w344 -> [w371 _]
        tunnel: w343 -> [w370 _]
        frame False {
        }
        frame True {
          n141 = global read "全局 时间2.vi" "时间2"() -> (w379:string)
          n142 = global read "全局 水样时间.vi" "时间"() -> (w373:string)
          n143 = Format Into String(format string="where 参数 = '%s' and 时间 between" ("condition"), w374) -> (resulting string=w378:string)  [unwired: 2 in, 1 out]
          n144 = Format Into String(format string="#%s#" ("初始字符串"), w373) -> (resulting string=w384:string)  [unwired: 2 in, 1 out]
          n145 = Format Into String(format string="#%s#" ("初始字符串"), w379) -> (resulting string=w380:string)  [unwired: 2 in, 1 out]
          n146 = Concatenate Strings(w378, w384, "and" ("字符串"), w380, " order by 时间 desc" ("字符串")) -> (w385:string)
          n147 = call "SQL查询.vi"("condition"=w385, "table输入"="仪器参数", "database"="database3.mdb") -> ("error out"=w386:errorcluster, "data"=w372:string[][])  [unwired: 5 in, 2 out]
        }
      }
      n148 = Get Date/Time In Seconds() -> (seconds since 1Jan1904=w360:timestamp)
      n149 = Format Date/Time String(time format string (%c)="%Y/%m/%d %H:%M:%S" ("时间格式字符串(%c)"), seconds (now)=w360) -> (date/time string=w361:string)  [unwired: 1 in]
      n150 = Search and Replace String(input string=w361, search string="." ("搜索字符串")) -> (result string=w357:string)  [unwired: 6 in, 3 out]
      n151 = Replace Array Subset(array=w363, new element=w357, index (row)=w358, index (col)=w358) -> (w356:string[][])
    }
    frame "报警信息", "报警信息存表" {
      # "时间"
      n152 = case shown="\"报警信息\", \"报警信息存表\", \"操作日志\", \"系统状态\"" w393 {
        tunnel: ["database1.mdb" ("database") "database3.mdb" ("database")] -> w404
        frame Default {
        }
        frame "报警信息", "报警信息存表", "操作日志", "系统状态" {
        }
      }
      n153 = case shown="\"环境参数\"" w393 {
        tunnel: [w454 "报警信息" ("table输入")] -> w394
        frame "环境参数" {
          n154 = local read "仪器日志参数"() -> (w454:string)
        }
        frame "报警信息", Default {
        }
      }
      n155 = case shown="\"环境参数\"" w389 {
        tunnel: [" order by 时间 desc" ("字符串") "" ("仪器日志参数")] -> w392
        frame "环境参数" {
        }
        frame "报警信息", Default {
        }
      }
      n156 = case shown="\"报警信息\"" w389 {
        tunnel: [w406 w409] -> w390
        tunnel: [w405 w408] -> w391
        tunnel: w388 -> [_ w410]
        frame "", Default {
          n157 = global read "全局 时间2.vi" "时间2"() -> (w405:string)
          n158 = global read "全局 水样时间.vi" "时间"() -> (w406:string)
        }
        frame "报警信息" {
          n159 = global read "全局 时间2.vi" "报警信息索引"() -> (w407:T4)
          n160 = case shown="\"氟化物\"" w410 {
            tunnel: [w411 w415 w418 w421 w424 w427 w430 w433 w436 w439 w442 w445 w448 w451] -> w408
            tunnel: [w412 w414 w416 w419 w422 w425 w428 w431 w434 w437 w440 w443 w446 w449] -> w409
            tunnel: w407 -> [_ w413 w417 w420 w423 w426 w429 w432 w435 w438 w441 w444 w447 w450]
            frame "假", Default {
              n161 = global read "全局 时间2.vi" "时间2"() -> (w411:string)
              n162 = global read "全局 水样时间.vi" "时间"() -> (w412:string)
            }
            frame "CODMn" {
              n163 = Unbundle By Name(w413) -> ("CODMn报警信息索引起始时间"=w414:string)
              n164 = global read "全局 时间2.vi" "时间2"() -> (w415:string)
            }
            frame "氨氮" {
              n165 = Unbundle By Name(w417) -> ("氨氮报警信息索引起始时间"=w416:string)
              n166 = global read "全局 时间2.vi" "时间2"() -> (w418:string)
            }
            frame "总磷" {
              n167 = Unbundle By Name(w420) -> ("总磷报警信息索引起始时间"=w419:string)
              n168 = global read "全局 时间2.vi" "时间2"() -> (w421:string)
            }
            frame "总氮" {
              n169 = Unbundle By Name(w423) -> ("总氮报警信息索引起始时间"=w422:string)
              n170 = global read "全局 时间2.vi" "时间2"() -> (w424:string)
            }
            frame "CODCr" {
              n171 = Unbundle By Name(w426) -> ("CODCr报警信息索引起始时间"=w425:string)
              n172 = global read "全局 时间2.vi" "时间2"() -> (w427:string)
            }
            frame "DO" {
              n173 = Unbundle By Name(w429) -> ("DO报警信息索引起始时间"=w428:string)
              n174 = global read "全局 时间2.vi" "时间2"() -> (w430:string)
            }
            frame "PH" {
              n175 = Unbundle By Name(w432) -> ("PH报警信息索引起始时间"=w431:string)
              n176 = global read "全局 时间2.vi" "时间2"() -> (w433:string)
            }
            frame "电导率" {
              n177 = Unbundle By Name(w435) -> ("比电导率报警信息索引起始时间"=w434:string)
              n178 = global read "全局 时间2.vi" "时间2"() -> (w436:string)
            }
            frame "水温" {
              n179 = Unbundle By Name(w438) -> ("水温报警信息索引起始时间"=w437:string)
              n180 = global read "全局 时间2.vi" "时间2"() -> (w439:string)
            }
            frame "浊度" {
              n181 = Unbundle By Name(w441) -> ("浊度报警信息索引起始时间"=w440:string)
              n182 = global read "全局 时间2.vi" "时间2"() -> (w442:string)
            }
            frame "叶绿素" {
              n183 = Unbundle By Name(w444) -> ("叶绿素报警信息索引起始时间"=w443:string)
              n184 = global read "全局 时间2.vi" "时间2"() -> (w445:string)
            }
            frame "系统" {
              n185 = Unbundle By Name(w447) -> ("系统报警信息索引起始时间"=w446:string)
              n186 = global read "全局 时间2.vi" "时间2"() -> (w448:string)
            }
            frame "氟化物" {
              n187 = Unbundle By Name(w450) -> ("氟化物报警信息索引起始时间"=w449:string)
              n188 = global read "全局 时间2.vi" "时间2"() -> (w451:string)
            }
          }
        }
      }
      n189 = case shown="\"报警信息\", 默认" w389 {
        tunnel: [w458 w462 "where 时间 between" ("condition")] -> w395
        tunnel: w388 -> [w457 w461 _]
        frame "报警信息", Default {
          n190 = call "数据库加密匹配 (子VI).vi"("输入参数"=w457) -> ("Encoded String"=w456:string)  [unwired: 10 in]
          n191 = Format Into String(format string="where 参数 = '%s' and 时间 between" ("condition"), w456) -> (resulting string=w458:string)  [unwired: 2 in, 1 out]
        }
        frame "环境参数" {
          n192 = call "数据库加密匹配 (子VI).vi"("输入参数"=w461) -> ("Encoded String"=w460:string)  [unwired: 10 in]
          n193 = Format Into String(format string="where 参数 = '%s' and 时间 between" ("condition"), w460) -> (resulting string=w462:string)  [unwired: 2 in, 1 out]
        }
        frame "报警信息存表" {
        }
      }
      n194 = Format Into String(format string="#%s#" ("初始字符串"), w391) -> (resulting string=w396:string)  [unwired: 2 in, 1 out]
      n195 = Format Into String(format string="#%s#" ("初始字符串"), w390) -> (resulting string=w400:string)  [unwired: 2 in, 1 out]
      n196 = Concatenate Strings(w395, w400, "and" ("字符串"), w396, w392) -> (w402:string)
      n197 = call "SQL查询.vi"("condition"=w402, "table输入"=w394, "database"=w404) -> ("error out"=w403:errorcluster, "data"=w401:string[][])  [unwired: 5 in, 2 out]
    }
    frame "提取报警信息" {
      w475 = 0 ("索引 (行)")
      # "时间"
      # "提取仪器状态"
      n198 = call "数据库加密匹配 (子VI).vi"("输入参数"=w478) -> ("Encoded String"=w468:string)  [unwired: 10 in]
      n199 = global read "全局 水样时间.vi" "时间"() -> (w484:string)
      n200 = global read "全局 时间2.vi" "时间2"() -> (w485:string)
      n201 = Format Into String(format string="where 参数 = '%s' and 时间 between" ("condition"), w468) -> (resulting string=w488:string)  [unwired: 2 in, 1 out]
      n202 = Format Into String(format string="#%s#" ("初始字符串"), w484) -> (resulting string=w493:string)  [unwired: 2 in, 1 out]
      n203 = Format Into String(format string="#%s#" ("初始字符串"), w485) -> (resulting string=w489:string)  [unwired: 2 in, 1 out]
      n204 = Concatenate Strings(w488, w493, "and" ("字符串"), w489, " order by 时间 desc" ("仪器日志参数")) -> (w494:string)
      n205 = call "SQL查询.vi"("condition"=w494, "columns"=string[] ["时间", "参数", "故障现象"], "table输入"="报警信息", "database"="database3.mdb") -> ("error out"=w495:errorcluster, "data"=w476:string[][])  [unwired: 4 in, 2 out]
      n206 = Index Array(array=w476, index (row)=w475, index (col)=w475) -> (element=w474:string)
      n207 = call "日期字符串格式至时间格式转换(子VI).vi"("data[0]"=w474) -> ("time stamp"=w472:timestamp)  [unwired: 10 in]
      n208 = Get Date/Time In Seconds() -> (seconds since 1Jan1904=w473:timestamp)
      n209 = Subtract(x=w473, y=w472) -> (x-y=w471:dbl)
      n210 = Format Date/Time String(time format string (%c)="%Y/%m/%d %H:%M:%S" ("时间格式字符串(%c)"), seconds (now)=w473) -> (date/time string=w481:string)  [unwired: 1 in]
      n211 = Greater Or Equal?(x=w471, y=86400.0) -> (x >= y?=w467:bool)
      n212 = Search and Replace String(input string=w481, search string="." ("搜索字符串")) -> (result string=w469:string)  [unwired: 6 in, 3 out]
      n213 = case shown="真" w467 {
        tunnel: [w499 w501] -> w479
        tunnel: w476 -> [w498 w503]
        tunnel: w469 -> [w497 w507]
        tunnel: w468 -> [_ w506]
        frame False {
          w500 = 0 ("索引 (行)")
          n214 = Replace Array Subset(array=w498, new element=w497, index (row)=w500, index (col)=w500) -> (w499:string[][])
        }
        frame True {
          n215 = Build Array(w507, w506, "无告警" ("元素")) -> (w502:string[])
          n216 = Replace Array Subset(array=w503, new element=w502, index (row)=0 ("索引 (行)")) -> (w501:string[][])  [unwired: 1 in]
        }
      }
    }
    frame "环境参数" {
      n217 = call "SQL查询.vi"("condition"=" order by 时间 desc" ("字符串"), "columns"=string[] ["时间", "电压", "室温", "湿度", "GPS经度", "GPS纬度"] ("columns输出 2"), "table输入"=w510, "database"="database1.mdb") -> ("error out"=w514:errorcluster, "columns输出"=w509:string[], "data"=w513:string[][])  [unwired: 4 in, 1 out]
    }
    frame Default {
      # "时间格式转换"
      n218 = local read "待发送数据"() -> (w516:string[][])
      n219 = call "数组时间戳格式化(子VI).vi"("待发送数据输入"=w516) -> ("待发送数据输出"=w515:string[][])  [unwired: 10 in]
    }
    frame "实时数据" {
      (unwired) " order by 时间 desc" ("字符串")
      w523 = "database1.mdb" ("database")
      # "上传本地时间点的实时数据"
      # "上传质控数据（空白测试，跨度核查，核查数据，平行样数据）"
      n220 = global read "全局 实时数据参数.vi" "实时数据参数"() -> (w519:string)
      n221 = case shown="\"空白测试\"" w519 {
        tunnel: [w574 w600 w629 w674] -> w538
        tunnel: w519 -> [w571 w595 _ w671]
        tunnel: [w572 w596 w626 w672] -> w534
        tunnel: w524 -> [_ w599 _ _]
        frame "水样测试" {
          n222 = call "数据库加密匹配 (子VI).vi"("输入参数"=w571) -> ("Encoded String"=w570:string)  [unwired: 10 in]
          n223 = call "数据库加密匹配 (子VI).vi"("输入参数"="N") -> ("Encoded String"=w568:string)  [unwired: 10 in]
          n224 = Get Date/Time In Seconds() -> (seconds since 1Jan1904=w582:timestamp)
          n225 = Format Date/Time String(time format string (%c)="%Y%m%d%H%M%S%3u" ("时间格式字符串(%c)"), seconds (now)=w582) -> (date/time string=w580:string)  [unwired: 1 in]
          n226 = local read "查询元素输入"() -> (w575:string)
          n227 = Replace Substring(2:8 ("长度（子字符串长度）"), 3:10 ("偏移量(0)"), 4:"0000" ("子字符串(\"\")"), 5:w580) -> (1:w576:string)  [unwired: 1 out]
          n228 = case shown="\"CODCr加标回收率\", \"CODMn加标回收率\", \"氨氮加标回收率\", \"总氮加标回收率\", \"总磷加标回收率\"" w575 {
            tunnel: w576 -> [w584 w587 _]
            tunnel: [w583 w588 w589] -> w574
            frame Default {
              n229 = Search and Replace String(input string=w584, search string="." ("搜索字符串")) -> (result string=w585:string)  [unwired: 6 in, 3 out]
              n230 = call "格式时间字符串.vi"("字符串"=w585) -> ("连接的字符串"=w583:string)  [unwired: 10 in]
            }
            frame "CODCr", "CODMn", "累积流量", "总氮", "总磷" {
              n231 = call "实时数据查询用2小时间的数据.vi"("字符串"=w587) -> ("连接的字符串"=w588:string)  [unwired: 10 in]
            }
            frame "CODCr加标回收率", "CODMn加标回收率", "氨氮加标回收率", "总氮加标回收率", "总磷加标回收率" {
              n232 = global read "全局 时间2.vi" "加标回收索引起始时间"() -> (w589:string)
            }
          }
          n233 = Format Into String(format string="where 测量模式 ='%s' and 数据类型 ='%s' and 时间 > " ("格式字符串"), w570, w568) -> (resulting string=w572:string)  [unwired: 2 in, 1 out]
        }
        frame "空白测试" {
          n234 = call "数据库加密匹配 (子VI).vi"("输入参数"=w595) -> ("Encoded String"=w594:string)  [unwired: 10 in]
          n235 = global read "全局 时间2.vi" "零点核查索引"() -> (w598:T5)
          n236 = case shown="\"挥发酚\"" w599 {
            tunnel: [w601 w603 w605 w607 w609 w612 w613 w615 w617 w619 w621] -> w600
            tunnel: w598 -> [w602 w604 w606 w608 w610 w611 w614 w616 w618 w620 _]
            frame "CODMn" {
              n237 = Unbundle By Name(w602) -> ("CODMn零点核查索引起始时间"=w601:string)
            }
            frame "CODCr" {
              n238 = Unbundle By Name(w604) -> ("CODCr零点核查索引起始时间"=w603:string)
            }
            frame "氨氮" {
              n239 = Unbundle By Name(w606) -> ("氨氮零点核查索引起始时间"=w605:string)
            }
            frame "总磷" {
              n240 = Unbundle By Name(w608) -> ("总磷零点核查索引起始时间"=w607:string)
            }
            frame "总氮" {
              n241 = Unbundle By Name(w610) -> ("总氮零点核查索引起始时间"=w609:string)
            }
            frame "亚硝酸盐" {
              n242 = Unbundle By Name(w611) -> ("亚硝酸盐零点核查索引起始时间"=w612:string)
            }
            frame "硫化物" {
              n243 = Unbundle By Name(w614) -> ("硫化物零点核查索引起始时间"=w613:string)
            }
            frame "ORP" {
              n244 = Unbundle By Name(w616) -> ("ORP零点核查索引起始时间"=w615:string)
            }
            frame "氟化物" {
              n245 = Unbundle By Name(w618) -> ("氟化物零点核查索引起始时间"=w617:string)
            }
            frame "挥发酚" {
              n246 = Unbundle By Name(w620) -> ("挥发酚零点核查索引起始时间"=w619:string)
            }
            frame "", Default {
              n247 = global read "全局 时间2.vi" "零点核查索引起始时间"() -> (w621:string)
            }
          }
          n248 = call "数据库加密匹配 (子VI).vi"("输入参数"="零点核查") -> ("Encoded String"=w592:string)  [unwired: 10 in]
          n249 = call "数据库加密匹配 (子VI).vi"("输入参数"="M") -> ("Encoded String"=w590:string)  [unwired: 10 in]
          n250 = Format Into String(format string="where (测量模式 ='%s' or 测量模式 = '%s') and 数据类型 <>'%s' and 时间 > " ("格式字符串"), w594, w592, w590) -> (resulting string=w596:string)  [unwired: 2 in, 1 out]
        }
        frame "核查数据" {
          n251 = global read "全局 时间2.vi" "标样核查索引"() -> (w628:T6)
          n252 = local read "查询元素输入"() -> (w630:string)
          n253 = case shown="\"挥发酚\"" w630 {
            tunnel: [w631 w633 w635 w637 w639 w641 w643 w645 w647 w649 w651 w653 w655 w657 w659 w661 w663 w665 w667] -> w629
            tunnel: w628 -> [w632 w634 w636 w638 w640 w642 w644 w646 w648 w650 w652 w654 w656 w658 w660 w662 w664 w666 _]
            frame "CODMn" {
              n254 = Unbundle By Name(w632) -> ("CODMn标样核查索引起始时间"=w631:string)
            }
            frame "CODCr" {
              n255 = Unbundle By Name(w634) -> ("CODCr标样核查索引起始时间"=w633:string)
            }
            frame "氨氮" {
              n256 = Unbundle By Name(w636) -> ("氨氮标样核查索引起始时间"=w635:string)
            }
            frame "总磷" {
              n257 = Unbundle By Name(w638) -> ("总磷标样核查索引起始时间"=w637:string)
            }
            frame "总氮" {
              n258 = Unbundle By Name(w640) -> ("总氮标样核查索引起始时间"=w639:string)
            }
            frame "DO" {
              n259 = Unbundle By Name(w642) -> ("DO标样核查索引起始时间"=w641:string)
            }
            frame "PH" {
              n260 = Unbundle By Name(w644) -> ("PH标样核查索引起始时间"=w643:string)
            }
            frame "比电导率" {
              n261 = Unbundle By Name(w646) -> ("比电导率标样核查索引起始时间"=w645:string)
            }
            frame "水温" {
              n262 = Unbundle By Name(w648) -> ("水温标样核查索引起始时间"=w647:string)
            }
            frame "浊度" {
              n263 = Unbundle By Name(w650) -> ("浊度标样核查索引起始时间"=w649:string)
            }
            frame "叶绿素a" {
              n264 = Unbundle By Name(w652) -> ("叶绿素a标样核查索引起始时间"=w651:string)
            }
            frame "藻密度" {
              n265 = Unbundle By Name(w654) -> ("藻密度标样核查索引起始时间"=w653:string)
            }
            frame "亚硝酸盐" {
              n266 = Unbundle By Name(w656) -> ("亚硝酸盐标样核查索引起始时间"=w655:string)
            }
            frame "硫化物" {
              n267 = Unbundle By Name(w658) -> ("硫化物标样核查索引起始时间"=w657:string)
            }
            frame "ORP" {
              n268 = Unbundle By Name(w660) -> ("ORP标样核查索引起始时间"=w659:string)
            }
            frame "氟化物" {
              n269 = Unbundle By Name(w662) -> ("氟化物标样核查索引起始时间"=w661:string)
            }
            frame "挥发酚" {
              n270 = Unbundle By Name(w664) -> ("挥发酚标样核查索引起始时间"=w663:string)
            }
            frame "氯化物" {
              n271 = Unbundle By Name(w666) -> ("氯化物标样核查索引起始时间"=w665:string)
            }
            frame "", Default {
              n272 = global read "全局 时间2.vi" "标样核查索引起始时间"() -> (w667:string)
            }
          }
          n273 = call "数据库加密匹配 (子VI).vi"("输入参数"="标样核查" ("实时数据参数")) -> ("Encoded String"=w622:string)  [unwired: 10 in]
          n274 = call "数据库加密匹配 (子VI).vi"("输入参数"="M") -> ("Encoded String"=w624:string)  [unwired: 10 in]
          n275 = Format Into String(format string="where 测量模式 ='%s' and 数据类型 <> '%s' and 时间 > " ("格式字符串"), w622, w624) -> (resulting string=w626:string)  [unwired: 2 in, 1 out]
        }
        frame "跨度核查", Default {
          n276 = call "数据库加密匹配 (子VI).vi"("输入参数"=w671) -> ("Encoded String"=w670:string)  [unwired: 10 in]
          n277 = call "数据库加密匹配 (子VI).vi"("输入参数"="M") -> ("Encoded String"=w668:string)  [unwired: 10 in]
          n278 = global read "全局 时间2.vi" "跨度核查索引"() -> (w676:T7)
          n279 = local read "查询元素输入"() -> (w675:string)
          n280 = case shown="\"挥发酚\"" w675 {
            tunnel: [w677 w679 w681 w683 w685 w688 w689 w691 w693 w695 w697] -> w674
            tunnel: w676 -> [w678 w680 w682 w684 w686 w687 w690 w692 w694 w696 _]
            frame "CODMn" {
              n281 = Unbundle By Name(w678) -> ("CODMn跨度核查索引起始时间"=w677:string)
            }
            frame "CODCr" {
              n282 = Unbundle By Name(w680) -> ("CODCr跨度核查索引起始时间"=w679:string)
            }
            frame "氨氮" {
              n283 = Unbundle By Name(w682) -> ("氨氮跨度核查索引起始时间"=w681:string)
            }
            frame "总磷" {
              n284 = Unbundle By Name(w684) -> ("总磷跨度核查索引起始时间"=w683:string)
            }
            frame "总氮" {
              n285 = Unbundle By Name(w686) -> ("总氮跨度核查索引起始时间"=w685:string)
            }
            frame "亚硝酸盐" {
              n286 = Unbundle By Name(w687) -> ("亚硝酸盐跨度核查索引起始时间"=w688:string)
            }
            frame "硫化物" {
              n287 = Unbundle By Name(w690) -> ("硫化物跨度核查索引起始时间"=w689:string)
            }
            frame "ORP" {
              n288 = Unbundle By Name(w692) -> ("ORP跨度核查索引起始时间"=w691:string)
            }
            frame "氟化物" {
              n289 = Unbundle By Name(w694) -> ("氟化物跨度核查索引起始时间"=w693:string)
            }
            frame "挥发酚" {
              n290 = Unbundle By Name(w696) -> ("挥发酚跨度核查索引起始时间"=w695:string)
            }
            frame "", Default {
              n291 = global read "全局 时间2.vi" "跨度核查索引起始时间"() -> (w697:string)
            }
          }
          n292 = Format Into String(format string="where 测量模式 ='%s' and 数据类型 <> '%s' and 时间 > " ("格式字符串"), w670, w668) -> (resulting string=w672:string)  [unwired: 2 in, 1 out]
        }
      }
      n293 = case shown="\"假\", 默认" w519 {
        tunnel: [string[] ["时间", "测量模式", "数据类型", "检测值", "单位", "数据标识", "标样参考值"] ("columns") string[] ["时间", "测量模式", "数据类型", "检测值", "单位", "数据标识", "标样参考值", "跨度值"] ("columns")] -> w529
        frame "假", Default {
        }
        frame "空白测试", "跨度核查" {
        }
      }
      n294 = global read "断电保存全局.vi" "数据发送延时时间/s"() -> (w528:i32)
      n295 = Get Date/Time In Seconds() -> (seconds since 1Jan1904=w527:timestamp)
      n296 = Subtract(x=w527, y=w528) -> (x-y=w526:timestamp)
      n297 = global read "断电保存全局.vi" "数据组合发送"() -> (w531:bool)
      n298 = Seconds To Date/Time(time stamp (now)=w526) -> (date time rec=w533:T8)  [unwired: 1 in]
      n299 = case shown="真" w531 {
        tunnel: w533 -> [w562 w567]
        tunnel: [w562 w566] -> w532
        frame False {
        }
        frame True {
          n300 = Unbundle By Name(w567) -> ("时"=w565:i32)
          n301 = Subtract(x=w565, y=2) -> (x-y=w563:i32)
          n302 = Bundle By Name(cluster=w567, "时"=w563) -> (w566:T8)
        }
      }
      n303 = Date/Time To Seconds(2:w532) -> (0:w537:timestamp)  [unwired: 1 in]
      n304 = Format Date/Time String(time format string (%c)="%Y/%m/%d %H:%M:%S" ("时间格式字符串(%c)"), seconds (now)=w537) -> (date/time string=w535:string)  [unwired: 1 in]
      n305 = Format Into String(format string="#%s#" ("初始字符串"), w538) -> (resulting string=w543:string)  [unwired: 2 in, 1 out]
      n306 = Format Into String(format string="#%s#" ("初始字符串"), w535) -> (resulting string=w540:string)  [unwired: 2 in, 1 out]
      n307 = Concatenate Strings(w534, w543, "and 时间 < " ("字符串"), w540, " order by 时间 asc" ("字符串")) -> (w522:string)
      n308 = call "SQL查询.vi"("condition"=w522, "columns"=w529, "table输入"=w524, "database"=w523) -> ("error out"=w525:errorcluster, "data"=w521:string[][])  [unwired: 4 in, 2 out]
      n309 = case shown="错误" w525 {
        selector: w525 -> [w544 _]
        tunnel: w519 -> [_ w552]
        tunnel: w524 -> [_ w551]
        tunnel: w523 -> [_ w550]
        tunnel: w522 -> [_ w549]
        tunnel: w521 -> [w545 w547]
        tunnel: [w545 w548] -> w520
        tunnel: [w544 w546] -> w518
        frame No Error {
        }
        frame Error {
          # "兼容旧数据库没有跨度值版本"
          n310 = case shown="\"空白测试\", \"跨度核查\"" w552 {
            tunnel: w551 -> [_ w558]
            tunnel: w550 -> [_ w557]
            tunnel: w549 -> [_ w556]
            tunnel: [w553 w555] -> w548
            tunnel: w547 -> [w553 _]
            tunnel: [_ w554] -> w546
            frame "假", Default {
            }
            frame "空白测试", "跨度核查" {
              n311 = call "SQL查询.vi"("condition"=w556, "columns"=string[] ["时间", "测量模式", "数据类型", "检测值", "单位", "数据标识", "标样参考值"], "table输入"=w558, "database"=w557) -> ("error out"=w554:errorcluster, "data"=w555:string[][])  [unwired: 4 in, 2 out]
            }
          }
        }
      }
      n312 = case shown="默认" w524 {
        tunnel: w524 -> [_ w700]
        tunnel: w522 -> [_ w699]
        tunnel: w520 -> [_ w698]
        frame Default {
        }
        frame "CODCr", "总氮", "总磷" {
          n313 = global write "全局 实时数据参数.vi" "data"(w698) -> ()
          n314 = global write "全局 实时数据参数.vi" "参数"(w700) -> ()
          n315 = global write "全局 实时数据参数.vi" "连接的字符串"(w699) -> ()
        }
      }
    }
    frame "加标回收" {
      w712 = "加标回收率" ("字符串")
      # "上传加标回收数据"
      n316 = call "数据库加密匹配 (子VI).vi"("输入参数"=w702) -> ("Encoded String"=w701:string)  [unwired: 10 in]
      n317 = global read "全局 数据发送重叠.vi" "掉线指示灯"() -> (w713:bool)
      n318 = case shown="假" w713 {
        tunnel: [w728 w744] -> w714
        frame False {
          n319 = global read "全局 时间2.vi" "加标回收索引"() -> (w734:T9)
          n320 = Unbundle By Name(w734) -> ("氨氮加标回收索引起始时间"=w733:string, "总磷加标回收索引起始时间"=w732:string, "总氮加标回收索引起始时间"=w731:string, "CODMn加标回收索引起始时间"=w730:string, "CODCr加标回收索引起始时间"=w729:string, "氟化物加标回收索引起始时间"=w727:string, "挥发酚加标回收索引起始时间"=w726:string)
          n321 = local read "查询元素输入"() -> (w735:string)
          n322 = case shown="\"挥发酚加标回收率\"" w735 {
            tunnel: [w736 w737 w738 w739 w740 w741 w742 w743] -> w728
            tunnel: w733 -> [_ _ w738 _ _ _ _ _]
            tunnel: w732 -> [_ _ _ w739 _ _ _ _]
            tunnel: w731 -> [_ _ _ _ w740 _ _ _]
            tunnel: w730 -> [w736 _ _ _ _ _ _ _]
            tunnel: w729 -> [_ w737 _ _ _ _ _ _]
            tunnel: w727 -> [_ _ _ _ _ w741 _ _]
            tunnel: w726 -> [_ _ _ _ _ _ w742 _]
            frame "CODMn加标回收率" {
            }
            frame "CODCr加标回收率" {
            }
            frame "氨氮加标回收率" {
            }
            frame "总磷加标回收率" {
            }
            frame "总氮加标回收率" {
            }
            frame "氟化物加标回收率" {
            }
            frame "挥发酚加标回收率" {
            }
            frame "", Default {
              n323 = global read "全局 时间2.vi" "加标回收索引起始时间"() -> (w743:string)
            }
          }
        }
        frame True {
          n324 = global read "全局 数据发送重叠.vi" "TCP掉线时间节点"() -> (w744:string)
        }
      }
      n325 = global read "断电保存全局.vi" "数据发送延时时间/s"() -> (w705:i32)
      n326 = Get Date/Time In Seconds() -> (seconds since 1Jan1904=w704:timestamp)
      n327 = Subtract(x=w704, y=w705) -> (x-y=w703:timestamp)
      n328 = Seconds To Date/Time(time stamp (now)=w703) -> (date time rec=w709:T8)  [unwired: 1 in]
      n329 = Date/Time To Seconds(2:w709) -> (0:w711:timestamp)  [unwired: 1 in]
      n330 = Format Date/Time String(time format string (%c)="%Y/%m/%d %H:%M:%S" ("时间格式字符串(%c)"), seconds (now)=w711) -> (date/time string=w708:string)  [unwired: 1 in]
      n331 = Format Into String(format string="#%s#" ("初始字符串"), w714) -> (resulting string=w725:string)  [unwired: 2 in, 1 out]
      n332 = Format Into String(format string="#%s#" ("初始字符串"), w708) -> (resulting string=w721:string)  [unwired: 2 in, 1 out]
      n333 = Concatenate Strings("where 参数 ='" ("condition"), w701, "' and 时间 > ", w725, "and 时间 < " ("字符串"), w721, " order by 时间 asc" ("字符串")) -> (w716:string)
      n334 = call "SQL查询.vi"("condition"=w716, "columns"=string[] ["时间", "参数", "加标前水样测试时间", "加标前水样浓度值", "加标后水样浓度值", "加标母液浓度值", "加标体积", "加标水杯定容体积", "加标回收率"], "table输入"=w712, "database"="database1.mdb") -> ("error out"=w717:errorcluster, "data"=w715:string[][])  [unwired: 4 in, 2 out]
      n335 = case shown="默认" w712 {
        tunnel: w712 -> [_ w747]
        tunnel: w716 -> [_ w746]
        tunnel: w715 -> [_ w745]
        frame Default {
        }
        frame "CODCr", "总氮", "总磷" {
          n336 = global write "全局 实时数据参数.vi" "data"(w745) -> ()
          n337 = global write "全局 实时数据参数.vi" "参数"(w747) -> ()
          n338 = global write "全局 实时数据参数.vi" "连接的字符串"(w746) -> ()
        }
      }
    }
    frame "平行样测试" {
      w759 = "平行样测试" ("字符串")
      # "上传本地时间点的实时数据"
      # "上传平行样数据"
      n339 = call "数据库加密匹配 (子VI).vi"("输入参数"=w749) -> ("Encoded String"=w748:string)  [unwired: 10 in]
      n340 = global read "全局 数据发送重叠.vi" "掉线指示灯"() -> (w760:bool)
      n341 = case shown="假" w760 {
        tunnel: [w785 w794] -> w761
        frame False {
          n342 = global read "全局 时间2.vi" "平行样索引"() -> (w783:T10)
          n343 = Unbundle By Name(w783) -> ("氨氮平行样索引起始时间"=w782:string, "总磷平行样索引起始时间"=w781:string, "总氮平行样索引起始时间"=w780:string, "CODMn平行样索引起始时间"=w779:string, "CODCr平行样索引起始时间"=w778:string, "氟化物平行样索引起始时间"=w777:string, "挥发酚平行样索引起始时间"=w776:string)
          n344 = local read "查询元素输入"() -> (w784:string)
          n345 = case shown="\"挥发酚\"" w784 {
            tunnel: [w786 w787 w788 w789 w790 w791 w792 w793] -> w785
            tunnel: w782 -> [_ _ w788 _ _ _ _ _]
            tunnel: w781 -> [_ _ _ w789 _ _ _ _]
            tunnel: w780 -> [_ _ _ _ w790 _ _ _]
            tunnel: w779 -> [w786 _ _ _ _ _ _ _]
            tunnel: w778 -> [_ w787 _ _ _ _ _ _]
            tunnel: w777 -> [_ _ _ _ _ w791 _ _]
            tunnel: w776 -> [_ _ _ _ _ _ w792 _]
            frame "CODMn" {
            }
            frame "CODCr" {
            }
            frame "氨氮" {
            }
            frame "总磷" {
            }
            frame "总氮" {
            }
            frame "氟化物" {
            }
            frame "挥发酚" {
            }
            frame "", Default {
              n346 = global read "全局 时间2.vi" "平行样索引起始时间"() -> (w793:string)
            }
          }
        }
        frame True {
          n347 = global read "全局 数据发送重叠.vi" "TCP掉线时间节点"() -> (w794:string)
        }
      }
      n348 = global read "断电保存全局.vi" "数据发送延时时间/s"() -> (w752:i32)
      n349 = Get Date/Time In Seconds() -> (seconds since 1Jan1904=w751:timestamp)
      n350 = Subtract(x=w751, y=w752) -> (x-y=w750:timestamp)
      n351 = Seconds To Date/Time(time stamp (now)=w750) -> (date time rec=w756:T8)  [unwired: 1 in]
      n352 = Date/Time To Seconds(2:w756) -> (0:w758:timestamp)  [unwired: 1 in]
      n353 = Format Date/Time String(time format string (%c)="%Y/%m/%d %H:%M:%S" ("时间格式字符串(%c)"), seconds (now)=w758) -> (date/time string=w755:string)  [unwired: 1 in]
      n354 = Format Into String(format string="#%s#" ("初始字符串"), w761) -> (resulting string=w775:string)  [unwired: 2 in, 1 out]
      n355 = Format Into String(format string="#%s#" ("初始字符串"), w755) -> (resulting string=w771:string)  [unwired: 2 in, 1 out]
      n356 = Concatenate Strings("where 参数 ='" ("condition"), w748, "' and 时间 > ", w775, "and 时间 < " ("字符串"), w771, " order by 时间 asc" ("字符串")) -> (w763:string)
      n357 = call "SQL查询.vi"("condition"=w763, "columns"=string[] ["时间", "参数", "第一次水样浓度值", "第二次水样测试时间", "第二次水样浓度值"], "table输入"=w759, "database"="database1.mdb") -> ("error out"=w765:errorcluster, "data"=w762:string[][])  [unwired: 4 in, 2 out]
      n358 = case shown="默认" w759 {
        tunnel: w759 -> [_ w797]
        tunnel: w763 -> [_ w796]
        tunnel: w762 -> [_ w795]
        frame Default {
        }
        frame "CODCr", "总氮", "总磷" {
          n359 = global write "全局 实时数据参数.vi" "data"(w795) -> ()
          n360 = global write "全局 实时数据参数.vi" "参数"(w797) -> ()
          n361 = global write "全局 实时数据参数.vi" "连接的字符串"(w796) -> ()
        }
      }
      n362 = case shown="假" FALSE {
        tunnel: [w799 w802] -> w767
        tunnel: w762 -> [w799 w801]
        tunnel: w765 -> [w798 w800]
        tunnel: [w798 w800] -> w764
        frame False {
        }
        frame True {
          # "数字字符串精度转换保留"
          n363 = Index Array(array=w801, index (col)=3 ("禁用的索引 (列)")) -> (element=w808:string[])  [unwired: 1 in]
          n364 = for {
            tunnel: w808 -> [w811] mode=indexing
            tunnel: [w810] -> w804 mode=indexing
            n365 = Fract/Exp String To Number(string=w811) -> (number=w812:dbl)  [unwired: 3 in, 1 out]
            n366 = Number To Fractional String(number=w812, precision (6)=i16 2 ("精度(6)")) -> (F-format string=w810:string)  [unwired: 2 in]
          }
          n367 = Delete From Array(array=w801, length=1 ("长度"), index (col)=3 ("禁用的索引 (列)")) -> (array with subset deleted=w805:string[][])  [unwired: 1 in, 1 out]
          n368 = Insert Into Array(array=w805, index (col)=3 ("禁用的索引 (列)"), new element=w804) -> (w802:string[][])  [unwired: 1 in]
        }
      }
    }
    frame "集成干预测试" {
      # "上传本地时间点的实时数据"
      # "上传集成干预数据"
      n369 = global read "全局 数据发送重叠.vi" "掉线指示灯"() -> (w827:bool)
      n370 = case shown="假" w827 {
        tunnel: [w851 w889] -> w828
        frame False {
          n371 = global read "全局 时间2.vi" "集成干预索引"() -> (w853:T11)
          n372 = local read "查询元素输入"() -> (w852:string)
          n373 = case shown="\"总磷\"" w852 {
            tunnel: [w854 w856 w858 w860 w862 w864 w866 w868 w870 w872 w874 w876 w878 w880 w882 w884 w886 w888] -> w851
            tunnel: w853 -> [w855 w857 w859 w861 w863 w865 w867 w869 w871 w873 w875 w877 w879 w881 w883 w885 w887 _]
            frame "CODMn" {
              n374 = Unbundle By Name(w855) -> ("CODMn集成干预索引起始时间"=w854:string)
            }
            frame "CODCr" {
              n375 = Unbundle By Name(w857) -> ("CODCr集成干预索引起始时间"=w856:string)
            }
            frame "氨氮" {
              n376 = Unbundle By Name(w859) -> ("氨氮集成干预索引起始时间"=w858:string)
            }
            frame "总磷" {
              n377 = Unbundle By Name(w861) -> ("总磷集成干预索引起始时间"=w860:string)
            }
            frame "总氮" {
              n378 = Unbundle By Name(w863) -> ("总氮集成干预索引起始时间"=w862:string)
            }
            frame "DO" {
              n379 = Unbundle By Name(w865) -> ("DO集成干预索引起始时间"=w864:string)
            }
            frame "PH" {
              n380 = Unbundle By Name(w867) -> ("PH集成干预索引起始时间"=w866:string)
            }
            frame "比电导率" {
              n381 = Unbundle By Name(w869) -> ("比电导率集成干预索引起始时间"=w868:string)
            }
            frame "水温" {
              n382 = Unbundle By Name(w871) -> ("水温集成干预索引起始时间"=w870:string)
            }
            frame "浊度" {
              n383 = Unbundle By Name(w873) -> ("浊度集成干预索引起始时间"=w872:string)
            }
            frame "叶绿素a" {
              n384 = Unbundle By Name(w875) -> ("叶绿素a集成干预索引起始时间"=w874:string)
            }
            frame "藻密度" {
              n385 = Unbundle By Name(w877) -> ("藻密度集成干预索引起始时间"=w876:string)
            }
            frame "亚硝酸盐" {
              n386 = Unbundle By Name(w879) -> ("亚硝酸盐集成干预索引起始时间"=w878:string)
            }
            frame "硫化物" {
              n387 = Unbundle By Name(w881) -> ("硫化物集成干预索引起始时间"=w880:string)
            }
            frame "ORP" {
              n388 = Unbundle By Name(w883) -> ("ORP集成干预索引起始时间"=w882:string)
            }
            frame "氟化物" {
              n389 = Unbundle By Name(w885) -> ("氟化物集成干预索引起始时间"=w884:string)
            }
            frame "挥发酚" {
              n390 = Unbundle By Name(w887) -> ("挥发酚集成干预索引起始时间"=w886:string)
            }
            frame "", Default {
              n391 = global read "全局 时间2.vi" "平行样索引起始时间"() -> (w888:string)
            }
          }
        }
        frame True {
          n392 = global read "全局 数据发送重叠.vi" "TCP掉线时间节点"() -> (w889:string)
        }
      }
      n393 = global read "断电保存全局.vi" "应用环境"() -> (w818:T3)
      n394 = case shown="\"STD\"" w818 {
        tunnel: w817 -> [w840 w850]
        tunnel: ["集成干预测试" ("字符串") w850] -> w816
        tunnel: [string[] ["时间", "参数", "集成干预测试浓度值", "集成干预前测试时间", "集成干预前测试浓度值"] ("columns") string[] ["时间", "测量模式", "数据类型", "检测值", "单位", "数据标识", "因子编码", "标样参考值"] ("columns")] -> w815
        tunnel: [w842 w849] -> w814
        frame "STD" {
          n395 = call "数据库加密匹配 (子VI).vi"("输入参数"=w840) -> ("Encoded String"=w839:string)  [unwired: 10 in]
          n396 = Concatenate Strings("where 参数 ='" ("condition"), w839) -> (w842:string)
        }
        frame "GB212", Default {
          n397 = call "数据库加密匹配 (子VI).vi"("输入参数"="集成干预测试" ("字符串")) -> ("Encoded String"=w845:string)  [unwired: 10 in]
          n398 = Concatenate Strings("where 测量模式 ='" ("condition"), w845) -> (w849:string)
        }
      }
      n399 = global read "断电保存全局.vi" "数据发送延时时间/s"() -> (w821:i32)
      n400 = Get Date/Time In Seconds() -> (seconds since 1Jan1904=w820:timestamp)
      n401 = Subtract(x=w820, y=w821) -> (x-y=w819:timestamp)
      n402 = Seconds To Date/Time(time stamp (now)=w819) -> (date time rec=w824:T8)  [unwired: 1 in]
      n403 = Date/Time To Seconds(2:w824) -> (0:w826:timestamp)  [unwired: 1 in]
      n404 = Format Date/Time String(time format string (%c)="%Y/%m/%d %H:%M:%S" ("时间格式字符串(%c)"), seconds (now)=w826) -> (date/time string=w823:string)  [unwired: 1 in]
      n405 = Format Into String(format string="#%s#" ("初始字符串"), w828) -> (resulting string=w838:string)  [unwired: 2 in, 1 out]
      n406 = Format Into String(format string="#%s#" ("初始字符串"), w823) -> (resulting string=w834:string)  [unwired: 2 in, 1 out]
      n407 = Concatenate Strings(w814, "' and 时间 > ", w838, "and 时间 < " ("字符串"), w834, " order by 时间 asc" ("字符串")) -> (w830:string)
      n408 = call "SQL查询.vi"("condition"=w830, "columns"=w815, "table输入"=w816, "database"="database1.mdb") -> ("error out"=w831:errorcluster, "data"=w829:string[][])  [unwired: 4 in, 2 out]
      n409 = case shown="\"CODCr\", \"总氮\", \"总磷\"" w816 {
        tunnel: w816 -> [_ w892]
        tunnel: w830 -> [_ w891]
        tunnel: w829 -> [_ w890]
        frame Default {
        }
        frame "CODCr", "总氮", "总磷" {
          n410 = global write "全局 实时数据参数.vi" "参数"(w892) -> ()
          n411 = global write "全局 实时数据参数.vi" "data"(w890) -> ()
          n412 = global write "全局 实时数据参数.vi" "连接的字符串"(w891) -> ()
        }
      }
    }
    frame "提取加标回收" {
      w897 = "加标回收率" ("字符串")
      # "上传本地时间点的实时数据"
      n413 = call "数据库加密匹配 (子VI).vi"("输入参数"=w894) -> ("Encoded String"=w893:string)  [unwired: 10 in]
      n414 = global read "全局 数据发送重叠.vi" "掉线指示灯"() -> (w898:bool)
      n415 = case shown="假" w898 {
        tunnel: [w914 w915] -> w899
        frame False {
          n416 = global read "起始时间.vi" "起始时间"() -> (w914:string)
        }
        frame True {
          n417 = global read "全局 数据发送重叠.vi" "TCP掉线时间节点"() -> (w915:string)
        }
      }
      n418 = global read "起始时间.vi" "结束时间"() -> (w896:string)
      n419 = Format Into String(format string="#%s#" ("初始字符串"), w899) -> (resulting string=w913:string)  [unwired: 2 in, 1 out]
      n420 = Format Into String(format string="#%s#" ("初始字符串"), w896) -> (resulting string=w909:string)  [unwired: 2 in, 1 out]
      n421 = Concatenate Strings("where 参数 ='" ("condition"), w893, "' and 时间 between ", w913, "and" ("字符串"), w909) -> (w901:string)
      n422 = call "SQL查询.vi"("condition"=w901, "columns"=string[] ["时间", "参数", "加标前水样测试时间", "加标前水样浓度值", "加标后水样浓度值", "加标母液浓度值", "加标体积", "加标水杯定容体积", "加标回收率"], "table输入"=w897, "database"="database1.mdb") -> ("error out"=w903:errorcluster, "data"=w900:string[][])  [unwired: 4 in, 2 out]
      n423 = case shown="\"CODCr\", \"总氮\", \"总磷\"" w897 {
        tunnel: w897 -> [_ w918]
        tunnel: w901 -> [_ w917]
        tunnel: w900 -> [_ w916]
        frame Default {
        }
        frame "CODCr", "总氮", "总磷" {
          n424 = global write "全局 实时数据参数.vi" "data"(w916) -> ()
          n425 = global write "全局 实时数据参数.vi" "参数"(w918) -> ()
          n426 = global write "全局 实时数据参数.vi" "连接的字符串"(w917) -> ()
        }
      }
      n427 = case shown="假" FALSE {
        tunnel: [w920 w923] -> w905
        tunnel: w900 -> [w920 w922]
        tunnel: w903 -> [w919 w921]
        tunnel: [w919 w921] -> w902
        frame False {
        }
        frame True {
          # "数字字符串精度转换保留"
          n428 = Index Array(array=w922, index (col)=3 ("禁用的索引 (列)")) -> (element=w929:string[])  [unwired: 1 in]
          n429 = for {
            tunnel: w929 -> [w932] mode=indexing
            tunnel: [w931] -> w925 mode=indexing
            n430 = Fract/Exp String To Number(string=w932) -> (number=w933:dbl)  [unwired: 3 in, 1 out]
            n431 = Number To Fractional String(number=w933, precision (6)=i16 2 ("精度(6)")) -> (F-format string=w931:string)  [unwired: 2 in]
          }
          n432 = Delete From Array(array=w922, length=1 ("长度"), index (col)=3 ("禁用的索引 (列)")) -> (array with subset deleted=w926:string[][])  [unwired: 1 in, 1 out]
          n433 = Insert Into Array(array=w926, index (col)=3 ("禁用的索引 (列)"), new element=w925) -> (w923:string[][])  [unwired: 1 in]
        }
      }
    }
    frame "提取平行样" {
      w939 = "平行样测试" ("字符串")
      # "上传本地时间点的实时数据"
      n434 = call "数据库加密匹配 (子VI).vi"("输入参数"=w936) -> ("Encoded String"=w935:string)  [unwired: 10 in]
      n435 = global read "全局 数据发送重叠.vi" "掉线指示灯"() -> (w940:bool)
      n436 = case shown="假" w940 {
        tunnel: [w956 w957] -> w941
        frame False {
          n437 = global read "起始时间.vi" "起始时间"() -> (w956:string)
        }
        frame True {
          n438 = global read "全局 数据发送重叠.vi" "TCP掉线时间节点"() -> (w957:string)
        }
      }
      n439 = global read "起始时间.vi" "结束时间"() -> (w938:string)
      n440 = Format Into String(format string="#%s#" ("初始字符串"), w941) -> (resulting string=w955:string)  [unwired: 2 in, 1 out]
      n441 = Format Into String(format string="#%s#" ("初始字符串"), w938) -> (resulting string=w951:string)  [unwired: 2 in, 1 out]
      n442 = Concatenate Strings("where 参数 ='" ("condition"), w935, "' and 时间 between ", w955, "and" ("字符串"), w951) -> (w943:string)
      n443 = call "SQL查询.vi"("condition"=w943, "columns"=string[] ["时间", "参数", "第一次水样浓度值", "第二次水样测试时间", "第二次水样浓度值"], "table输入"=w939, "database"="database1.mdb") -> ("error out"=w945:errorcluster, "data"=w942:string[][])  [unwired: 4 in, 2 out]
      n444 = case shown="\"CODCr\", \"总氮\", \"总磷\"" w939 {
        tunnel: w939 -> [_ w960]
        tunnel: w943 -> [_ w959]
        tunnel: w942 -> [_ w958]
        frame Default {
        }
        frame "CODCr", "总氮", "总磷" {
          n445 = global write "全局 实时数据参数.vi" "data"(w958) -> ()
          n446 = global write "全局 实时数据参数.vi" "参数"(w960) -> ()
          n447 = global write "全局 实时数据参数.vi" "连接的字符串"(w959) -> ()
        }
      }
      n448 = case shown="假" FALSE {
        tunnel: [w962 w965] -> w947
        tunnel: w942 -> [w962 w964]
        tunnel: w945 -> [w961 w963]
        tunnel: [w961 w963] -> w944
        frame False {
        }
        frame True {
          # "数字字符串精度转换保留"
          n449 = Index Array(array=w964, index (col)=3 ("禁用的索引 (列)")) -> (element=w971:string[])  [unwired: 1 in]
          n450 = for {
            tunnel: w971 -> [w974] mode=indexing
            tunnel: [w973] -> w967 mode=indexing
            n451 = Fract/Exp String To Number(string=w974) -> (number=w975:dbl)  [unwired: 3 in, 1 out]
            n452 = Number To Fractional String(number=w975, precision (6)=i16 2 ("精度(6)")) -> (F-format string=w973:string)  [unwired: 2 in]
          }
          n453 = Delete From Array(array=w964, length=1 ("长度"), index (col)=3 ("禁用的索引 (列)")) -> (array with subset deleted=w968:string[][])  [unwired: 1 in, 1 out]
          n454 = Insert Into Array(array=w968, index (col)=3 ("禁用的索引 (列)"), new element=w967) -> (w965:string[][])  [unwired: 1 in]
        }
      }
    }
    frame "提取集成干预" {
      # "上传本地时间点的实时数据"
      n455 = global read "断电保存全局.vi" "应用环境"() -> (w981:T3)
      n456 = case shown="\"GB212\", 默认" w981 {
        tunnel: w977 -> [w999 w1009]
        tunnel: ["集成干预测试" ("字符串") w1009] -> w979
        tunnel: [string[] ["时间", "参数", "集成干预测试浓度值", "集成干预前测试时间", "集成干预前测试浓度值"] ("columns") string[] ["时间", "测量模式", "数据类型", "检测值", "单位", "数据标识", "因子编码", "标样参考值"] ("columns")] -> w980
        tunnel: [w1001 w1008] -> w978
        frame "STD" {
          n457 = call "数据库加密匹配 (子VI).vi"("输入参数"=w999) -> ("Encoded String"=w998:string)  [unwired: 10 in]
          n458 = Concatenate Strings("where 参数 ='" ("condition"), w998) -> (w1001:string)
        }
        frame "GB212", Default {
          n459 = call "数据库加密匹配 (子VI).vi"("输入参数"="集成干预测试" ("字符串")) -> ("Encoded String"=w1004:string)  [unwired: 10 in]
          n460 = Concatenate Strings("where 测量模式 ='" ("condition"), w1004) -> (w1008:string)
        }
      }
      n461 = global read "全局 数据发送重叠.vi" "掉线指示灯"() -> (w983:bool)
      n462 = case shown="假" w983 {
        tunnel: [w1010 w1011] -> w984
        frame False {
          n463 = global read "起始时间.vi" "起始时间"() -> (w1010:string)
        }
        frame True {
          n464 = global read "全局 数据发送重叠.vi" "TCP掉线时间节点"() -> (w1011:string)
        }
      }
      n465 = global read "起始时间.vi" "结束时间"() -> (w982:string)
      n466 = Format Into String(format string="#%s#" ("初始字符串"), w984) -> (resulting string=w997:string)  [unwired: 2 in, 1 out]
      n467 = Format Into String(format string="#%s#" ("初始字符串"), w982) -> (resulting string=w993:string)  [unwired: 2 in, 1 out]
      n468 = Concatenate Strings(w978, "' and 时间 between ", w997, "and" ("字符串"), w993) -> (w986:string)
      n469 = call "SQL查询.vi"("condition"=w986, "columns"=w980, "table输入"=w979, "database"="database1.mdb") -> ("error out"=w988:errorcluster, "data"=w985:string[][])  [unwired: 4 in, 2 out]
      n470 = case shown="\"CODCr\", \"总氮\", \"总磷\"" w979 {
        tunnel: w979 -> [_ w1014]
        tunnel: w986 -> [_ w1013]
        tunnel: w985 -> [_ w1012]
        frame Default {
        }
        frame "CODCr", "总氮", "总磷" {
          n471 = global write "全局 实时数据参数.vi" "data"(w1012) -> ()
          n472 = global write "全局 实时数据参数.vi" "参数"(w1014) -> ()
          n473 = global write "全局 实时数据参数.vi" "连接的字符串"(w1013) -> ()
        }
      }
      n474 = case shown="假" FALSE {
        tunnel: [w1016 w1019] -> w990
        tunnel: w985 -> [w1016 w1018]
        tunnel: w988 -> [w1015 w1017]
        tunnel: [w1015 w1017] -> w987
        frame False {
        }
        frame True {
          # "数字字符串精度转换保留"
          n475 = Index Array(array=w1018, index (col)=3 ("禁用的索引 (列)")) -> (element=w1025:string[])  [unwired: 1 in]
          n476 = for {
            tunnel: w1025 -> [w1028] mode=indexing
            tunnel: [w1027] -> w1021 mode=indexing
            n477 = Fract/Exp String To Number(string=w1028) -> (number=w1029:dbl)  [unwired: 3 in, 1 out]
            n478 = Number To Fractional String(number=w1029, precision (6)=i16 2 ("精度(6)")) -> (F-format string=w1027:string)  [unwired: 2 in]
          }
          n479 = Delete From Array(array=w1018, length=1 ("长度"), index (col)=3 ("禁用的索引 (列)")) -> (array with subset deleted=w1022:string[][])  [unwired: 1 in, 1 out]
          n480 = Insert Into Array(array=w1022, index (col)=3 ("禁用的索引 (列)"), new element=w1021) -> (w1019:string[][])  [unwired: 1 in]
        }
      }
    }
    frame "提取实时数据" {
      # "上传给定时间段之间的实时数据"
      n481 = global read "全局 实时数据参数.vi" "实时数据参数"() -> (w1032:string)
      n482 = call "数据库加密匹配 (子VI).vi"("输入参数"=w1032) -> ("Encoded String"=w1031:string)  [unwired: 10 in]
      n483 = global read "起始时间.vi" "起始时间"() -> (w1043:string)
      n484 = global read "起始时间.vi" "结束时间"() -> (w1042:string)
      n485 = Format Into String(format string="#%s#" ("初始字符串"), w1043) -> (resulting string=w1050:string)  [unwired: 2 in, 1 out]
      n486 = Format Into String(format string="#%s#" ("初始字符串"), w1042) -> (resulting string=w1044:string)  [unwired: 2 in, 1 out]
      n487 = Concatenate Strings("where 测量模式 ='" ("condition"), w1031, "' and 时间 between ", w1050, "and" ("字符串"), w1044) -> (w1048:string)
      n488 = call "SQL查询.vi"("condition"=w1048, "columns"=string[] ["时间", "测量模式", "数据类型", "检测值", "单位", "数据标识", "标样参考值"], "table输入"=w1034, "database"="database1.mdb") -> ("error out"=w1039:errorcluster, "data"=w1041:string[][])  [unwired: 4 in, 2 out]
      n489 = case shown="假" FALSE {
        tunnel: w1041 -> [w1052 w1060]
        tunnel: [w1052 w1054] -> w1040
        tunnel: w1039 -> [w1051 w1053]
        tunnel: [w1051 w1053] -> w1038
        frame False {
        }
        frame True {
          # "数字字符串精度转换保留"
          n490 = Index Array(array=w1060, index (col)=3 ("禁用的索引 (列)")) -> (element=w1061:string[])  [unwired: 1 in]
          n491 = for {
            tunnel: w1061 -> [w1064] mode=indexing
            tunnel: [w1063] -> w1056 mode=indexing
            n492 = Fract/Exp String To Number(string=w1064) -> (number=w1065:dbl)  [unwired: 3 in, 1 out]
            n493 = Number To Fractional String(number=w1065, precision (6)=i16 2 ("精度(6)")) -> (F-format string=w1063:string)  [unwired: 2 in]
          }
          n494 = Delete From Array(array=w1060, length=1 ("长度"), index (col)=3 ("禁用的索引 (列)")) -> (array with subset deleted=w1057:string[][])  [unwired: 1 in, 1 out]
          n495 = Insert Into Array(array=w1057, index (col)=3 ("禁用的索引 (列)"), new element=w1056) -> (w1054:string[][])  [unwired: 1 in]
        }
      }
    }
  }
  "待发送数据" <- w1
  "columns输出" <- w2
  n496 = call <vilib>:"Clear Errors.vi"("error in (no error)"=w8) -> ("error out"=→"error out":errorcluster)  [unwired: 5 in, 1 out]
  n497 = Index Array(array=w1, index (row)=0 ("索引 (行)")) -> (element=→"待发送第一条数据":string[])  [unwired: 1 in]
